vi "Striptest.vi"(1 "Simulation?":bool) -> ()   [LabVIEW 2013]
uses:
  InstrControl/SupplyControl/SupplyControl.lvclass
  InstrControl/Switching/Switching.lvclass
  InstrControl/ProbeStationControl/ProbeStationControl.lvclass
  InstrControl/LCRControl/LCRControl.lvclass
  general_VIs/globals/QC_MeasurementSetup.vi
  striptest/ProbePlan/ProbePlanParams.vi
  general_VIs/globals/QC_RunInformation.vi
  InstrControl/InstrumentSetup.vi
  <vilib>/regexp/Match Regular Expression.xnode
  InstrControl/InstrControl.lvclass
  InstrControl/ArduinoControl/ArduinoControl.lvclass
  <vilib>/Analysis/NI_AALBase.lvlib
panel:
  out "Tab Control":enum32{"Striptest Setup", "Striptest"}(tab)
  in  "Bias Voltage [V]":dbl=-150.0 format="%.1f"
  in  "Frequency [Hz] Setup":i32=500 caption="Frequency [Hz]" format="%#.3p"
  in  "Minimum fraction\nof good strips":dbl=-500.0 format="%.1g"
  in  "Quit":bool
  in  "Continue":bool
  in  "Measurement Configurations":bool
  in  "Pinholes Y/N":bool=TRUE
  in  "Capacitance Y/N":bool=TRUE
  in  "Resistance Y/N":bool=TRUE
  in  "Striptest SMU":string(combo)="Keithley 2410"
  in  "LCR Meter":string(combo)="WayneKerr 6440B"
  in  "Temperature":enum16{"Read Arduino", "Enter manually"}(ring)
  in  "Bias Supply":string(combo)="Keithley 2410"
  in  "Hardware Configurations":bool
  in  "DB Serial No. IN:":string caption="DB Serial No.:"
  in  "User:":string(combo)="Christoph"
  in  "Batch No. IN:":string caption="Batch No.:"
  in  "Device Category IN:":string(combo)="Short Strip" caption="Device Category:"
  in  "Sensor Serial No. IN:":string caption="Sensor Serial No.:"
  in  "From4":u16(ring)
  in  "From3":u16(ring)
  in  "From2":u16(ring)
  in  "From 1":u16(ring) caption="From"
  in  "To4":u16(ring)
  in  "To3":u16(ring)
  in  "To2":u16(ring)
  in  "To 1":u16(ring) caption="To"
  out "Region 1":string caption="Region"
  out "Region2":string
  out "Region3":string
  out "Region4":string
  in  "Enable1":bool
  in  "Enable4":bool
  in  "Enable2":bool
  in  "Enable3":bool
  in  "Pinhole Parameters IN":T1={"Base Voltage"=10.0, "Base Ramp [V/step]"=10.0, "Base Step [ms]"=1000, "High Voltage"=100.0, "High Ramp [V/step]"=100.0, "High Step [ms]"=1000} caption="Pinhole Measurement Parameters"
  in  "Manufacturer:":string(combo)="Hamamatsu"
  in  "Auto ReCheck":bool
  in  "Thresholds:":T2={"Current [nA]"=200.0, "Ccoupl Lo [pF/cm]"=20.0, "Ccoupl Hi [pF/cm]"=33.0, "Rbias Lo [MW]"=1.0, "Rbias Hi [MW]"=2.0}
  in  "Rolling\nCurrent Readout":bool=TRUE
  in  "settling\ndelay [ms]":i32=50
  in  "Pinhole Parameters":T1={"Base Voltage"=10.0, "Base Ramp [V/step]"=10.0, "Base Step [ms]"=1000, "High Voltage"=100.0, "High Ramp [V/step]"=100.0, "High Step [ms]"=1000}
  out "Bias On/Off:":bool
  in  "Auto quit &\nswitch off bias":bool
  out "Sensor No.:":string
  out "Device Category:":string
  out "DB Serial No.:":string
  out "Initiated:":string
  in  "ReCheck":bool
  in  "Save Data":bool
  in  "Abort":bool
  in  "Quit w/o saving":bool
  out "Probing Region:":string
  out "Probe Point:":string
  out "Current [nA]:":dbl
  out "Capacitance [pF]:":dbl
  out "Reistance [MW]:":dbl
  out "Last Probe at:":string
  out "Run Duration:":string
  out "Estimated Completion:":string
  out "Status:":string
  out "Probe Card Channels":i32=32
  in  "Show:":u16(ring)
  out "Defects":i32[][](graph)
  out "% OK:":dbl
  out "# total defects:":i32
  out "# probed":i32
  in  "Display Stats":bool=TRUE
  out "Bad Strip List":i32[](array[numeric])
  out "defect type array":i32[](array[numeric])
  out "Resistance [MW]":cluster{u32, i32, "Array OUT":dbl[]}(graph)
  out "Capacitance [pF]":cluster{u32, i32, "Array OUT":dbl[]}(graph)
  out "Current [nA]":cluster{u32, i32, "Array OUT":dbl[]}(graph)
  out "Current Reference 100V":dbl[](array[numeric])
  out "Current Reference 10V":dbl[](array[numeric])
  out "Single Needle":bool
  out "Z profile":i32[][](array[numeric])
  out "Start Temperature [°C]":dbl
  out "Last Temperature [°C]":dbl
  out "disabled channels":i32[](array[numeric])
  out "Module failed/passed":bool
  out "probe points per region":i32[](array[numeric])
  out "min scale array":i32[](array[numeric])
  out "max scale array":i32[](array[numeric])
  out "total strip number":u32
  out "Region Indices":i32[](array[numeric])
  out "Current Bias Voltage [V]":dbl
  out "Temperature Progression":T3
  # "University of \nCambridge"
  # "Sensor QC: Striptest"
  # "Current [nA]"
  # "Statistical information:"
  # "Pinholes:"
  # "Capacitance [pF]"
  # "Punchthroughs:"
  # "Shorts:"
  # "Opens:"
  # "Rpoly:"
  # "Resistance [MW]"
  # "Implant:"
  # "Current segment:"
  # "Ok  Pinhole at base  Pinhole after ramp  Short  Open  Rbias"
  # "Probe Range"
  # "Measurement Configuration"
  # "Hardware"
  # "DUT Description"
  # "Tests Included"
  # "Current status:"
  # "Measurement parameters:"
  # "DUT & Test Description:"
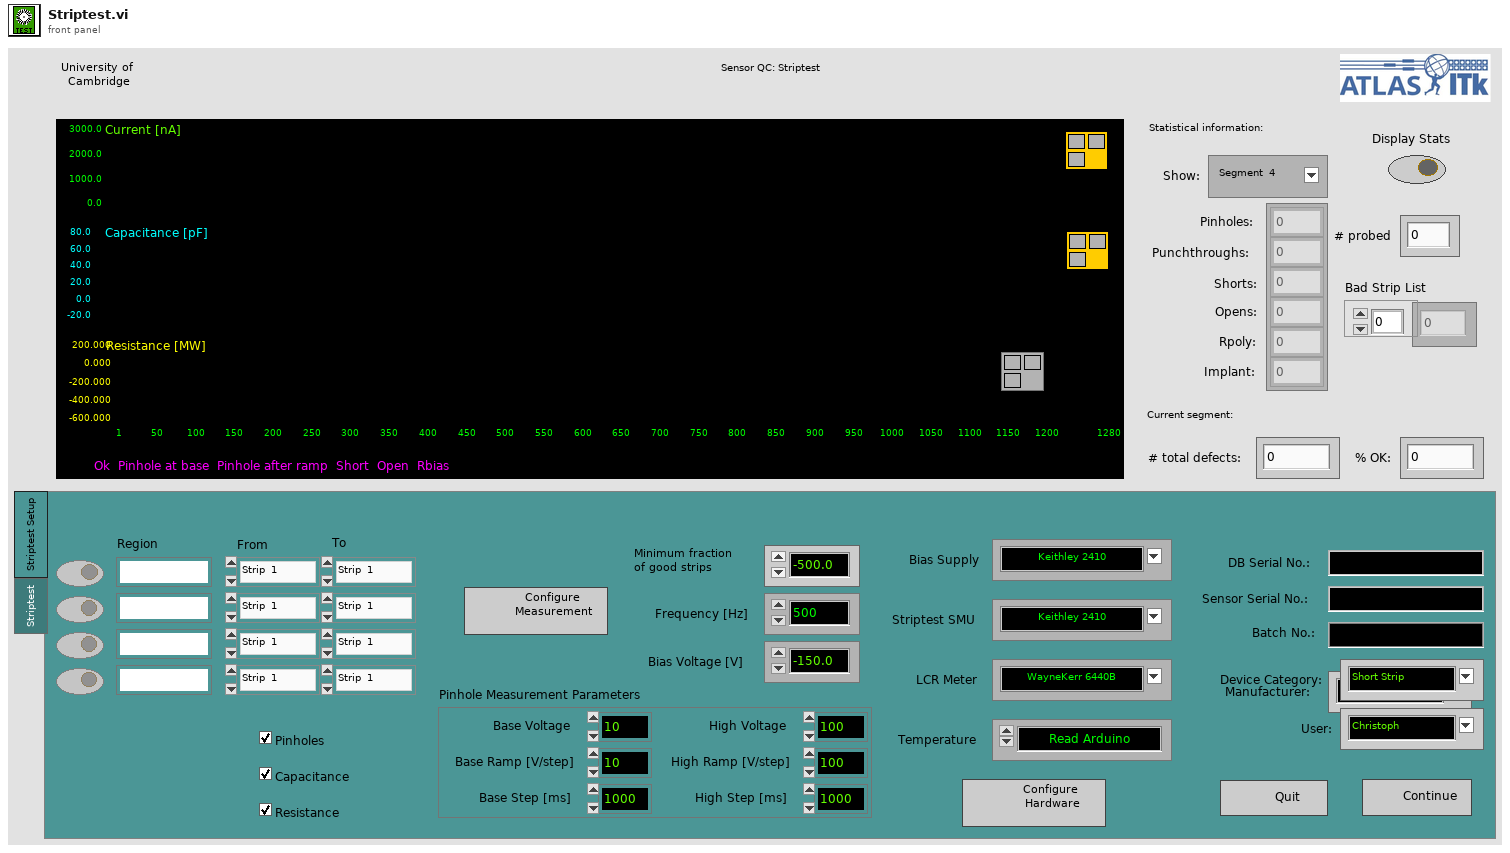
[diagram p1: front panel]
types:
  T1 = cluster{"Base Voltage":dbl, "Base Ramp [V/step]":dbl, "Base Step [ms]":i32, "High Voltage":dbl, "High Ramp [V/step]":dbl, "High Step [ms]":i32}
  T2 = cluster{"Current [nA]":dbl, "Ccoupl Lo [pF/cm]":dbl, "Ccoupl Hi [pF/cm]":dbl, "Rbias Lo [MW]":dbl, "Rbias Hi [MW]":dbl}
  T3 = cluster{"Time Array":string[], "Temperature Array [°C]":dbl[], "Humidity Array [RH %]":dbl[]}
  T4 = enum16{"Supply", "LCR", "Multimeter", "Switching"}
  T5 = enum16{"Reset", "Ground", "Striptest SMU", "Striptest LCR", "IV", "CV", "Interstrip Cap", "Interstrip Res"}
  T6 = enum16{"Reference measurement", "Baseline correcetion 10V", "Baseline correcetion 100V", "Nothing"}
  T7 = cluster{"Bias Supply":refnum<class "SupplyControl.lvclass">, "SMU":refnum<class "SupplyControl.lvclass">, "LCR":refnum<class "LCRControl.lvclass">, "Probe Card Channels":i32, "Bias Voltage [V]":dbl, "First strip":i32, "Last strip":i32, "Base Voltage [V]":dbl, "Base Ramp Step [V]":dbl, "Base Ramp Interval [ms]":u32, "High Voltage [V]":dbl, "High Ramp Step [V]":dbl, "High Ramp Interval [ms]":u32, "AC frequency [Hz]":i32, "AC amplitude [V]":dbl, "RC Configuration":u16, "Single Needle":bool, "Temperature Readout":enum16{"Read Arduino", "Enter manually"}, "Arduino":refnum<class "ArduinoControl.lvclass">, "Fraction of good strips [%]":dbl, "ProbeStation":refnum<class "ProbeStationControl.lvclass">, "Switching":refnum<class "Switching.lvclass">, "Matrix used?":bool, "Matrix X Channels":cluster{"Bias Supply / SMU LO":i32, "Bias Supply / SMU HI":i32, "CV Box LO":i32, "CV Box HI":i32, "CV Box LO IN":i32, "CV Box HI IN":i32, "Volt meter LO":i32, "Volt meter HI":i32, "Mux1 C1":i32, "Mux1 C2":i32, "Mux2 C1":i32, "Mux2 C2":i32}, "Pinholes Y/N":bool, "Capacitance Y/N":bool, "Resistance Y/N":bool, "Bias Supply Name":string, "SMU Name":string, "LCR Name":string}
  T8 = cluster{"Sensor Serial No.:":string, "Wafer Serial No.:":string, "Batch:":string, "Manufacturer:":string, "Device Category:":string, "Database Serial No.:":string, "Date Initiated:":string, "Time Initiated:":string, "Test":string, "Instruments used:":string, "Probeplan used:":string, "End of Run comment:":string, "User:":string}
  T9 = cluster{"Institute":string, "Manufacturers":string[], "Devices":string[], "Serialnumbers Lookup DB":string, "Data directory":string, "Backup & screenshot directory":string, "List of known users":string[]}
  T10 = cluster{"Strip Number OUT":i32, "X0":i32, "Y0":i32, "X1":i32, "Y1":i32, "Xref":dbl, "Yref":dbl, "ProbePlan type":u32, "Inner pads offset":ext, "Outer pads offset":ext, "l_inner":ext, "l_outer":ext, "strip numbering":u16, "Device Orientation":ext, "Stagger offset":i32, "Yoffset":dbl, "Strip pitch":dbl, "Fiducail separation":dbl, "Radius":ext, "Relative strip angles":dbl, "Probeplan description":string, "ProbePlan array":cluster{"Region":string, "ProbePoints":cluster{"X":dbl, "Y":dbl, "Label":string, "CardViable?":bool}[]}[], "Test ProbePoints":cluster{"Regions Enabled":bool[], "From index":u32[], "To index":u32[]}}
  T11 = cluster{"Region":string, "ProbePoints":cluster{"X":dbl, "Y":dbl, "Label":string, "CardViable?":bool}[]}[]
  T12 = cluster{"VISA address":refnum<visa-resource-name>, "T sensor":enum16{"SHT", "DS"}, "Arduino":refnum<class "ArduinoControl.lvclass">}
  T13 = cluster{"X":dbl, "Y":dbl, "Label":string, "CardViable?":bool}[]
  T14 = cluster{"X":dbl, "Y":dbl, "Label":string, "CardViable?":bool}
  T15 = cluster{"pass Rate in %":dbl, "Bad channel list":i32[], "No of bad strips":i32, "Defect description list":i32[], "Number of defects per category":i32[], "Defect lists":string[], "No of channels":i32, "Defect Flag array OUT":i32[][]}
  T16 = cluster{"Hi Cap":dbl, "Lo Cap":dbl, "Current threshold":dbl, "Lo R":dbl, "Hi R":dbl}
  T17 = enum16{"Reset", "Read Array", "Read Element", "Write Element", "Write Array", "Add Element", "Add Array"}
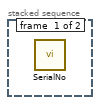
[diagram p2: hidden frame]
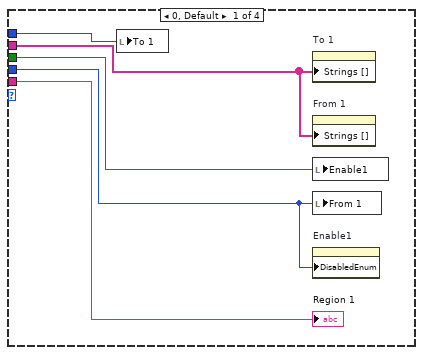
[diagram p3: hidden frame]
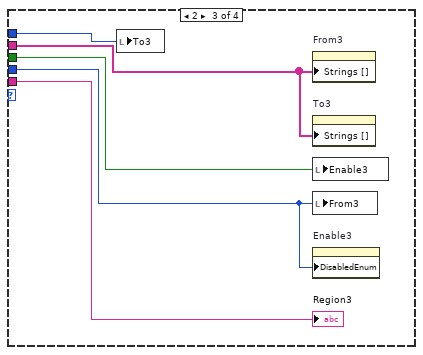
[diagram p4: hidden frame]
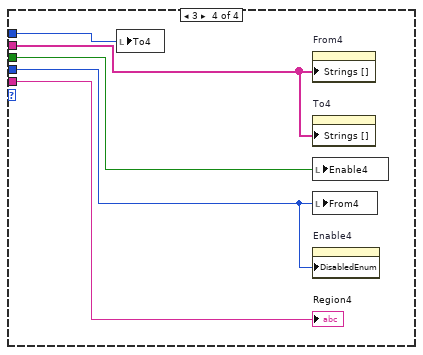
[diagram p5: hidden frame]
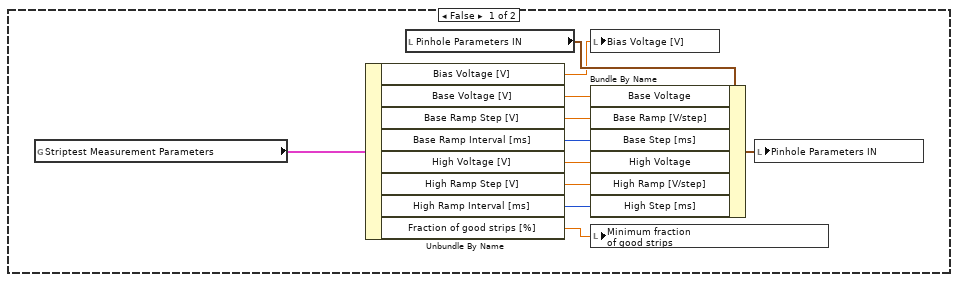
[diagram p7: hidden frame]
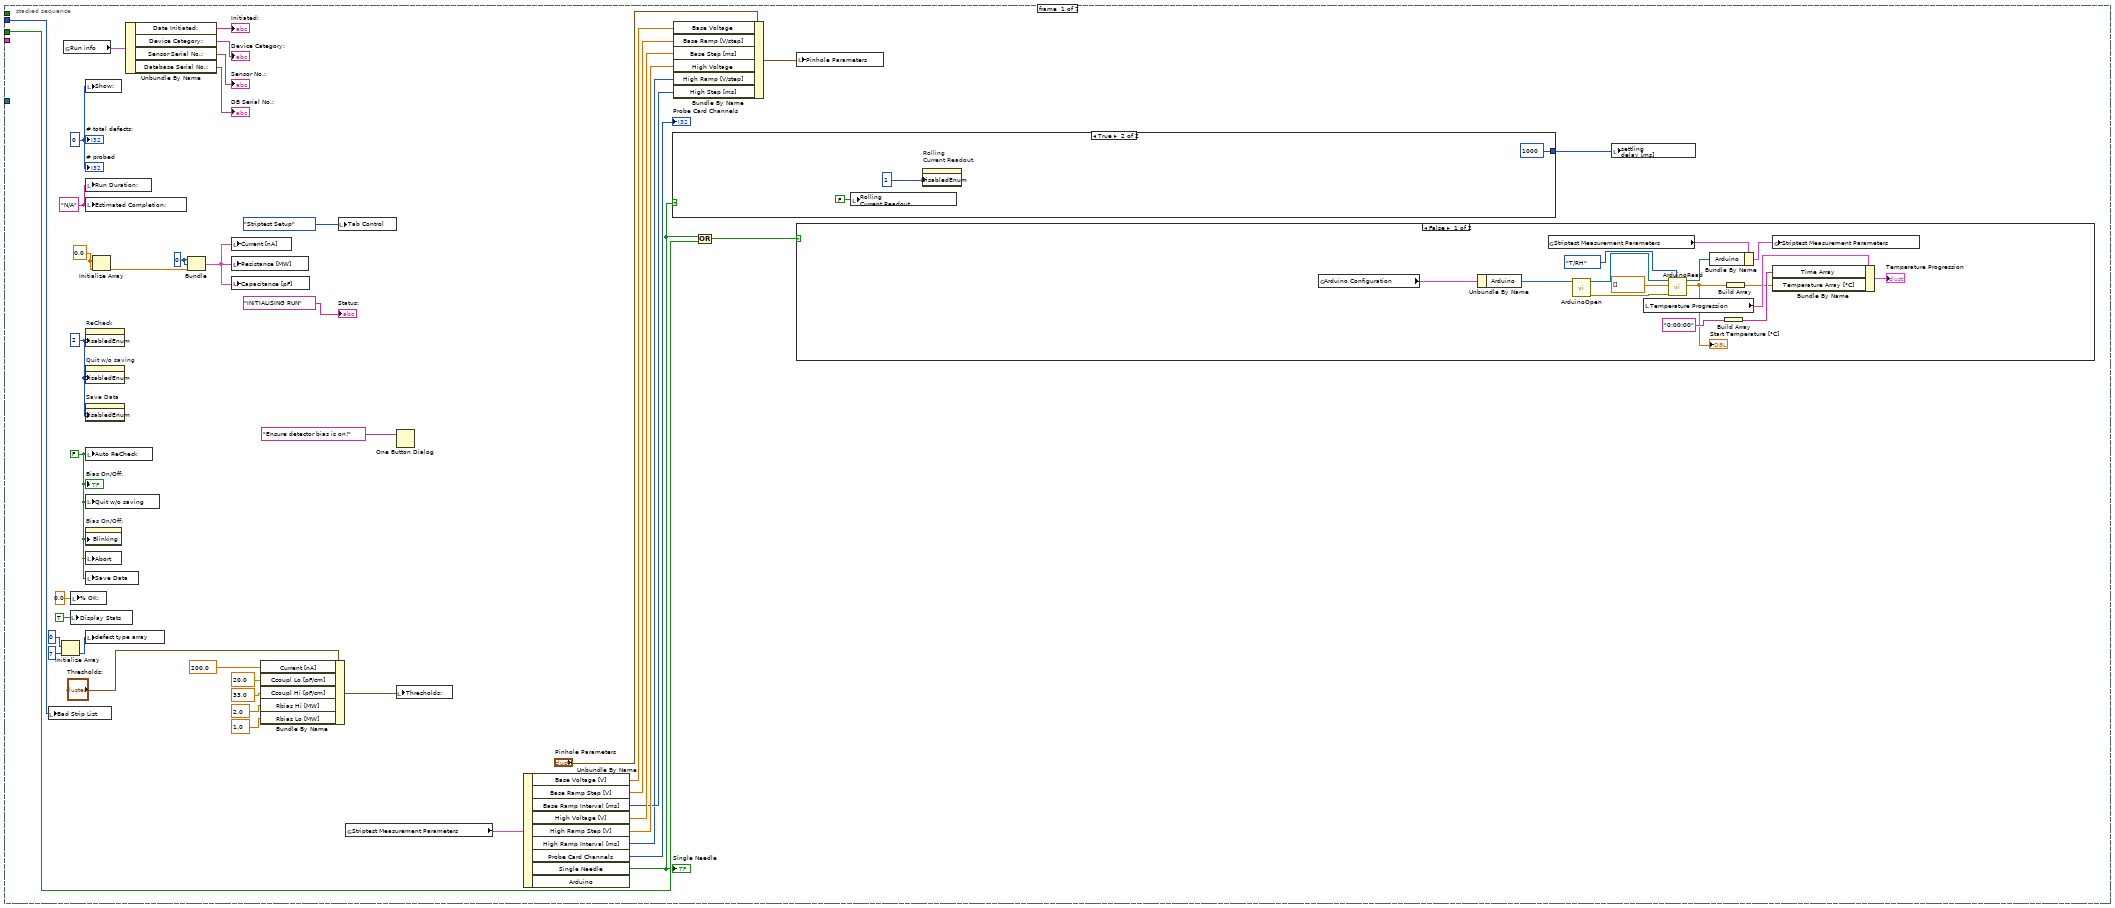
[diagram p10: hidden frame]
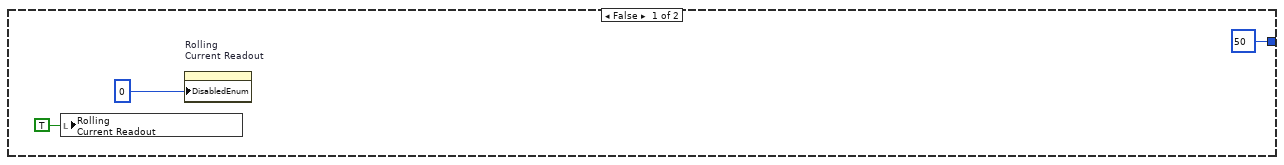
[diagram p11: hidden frame]
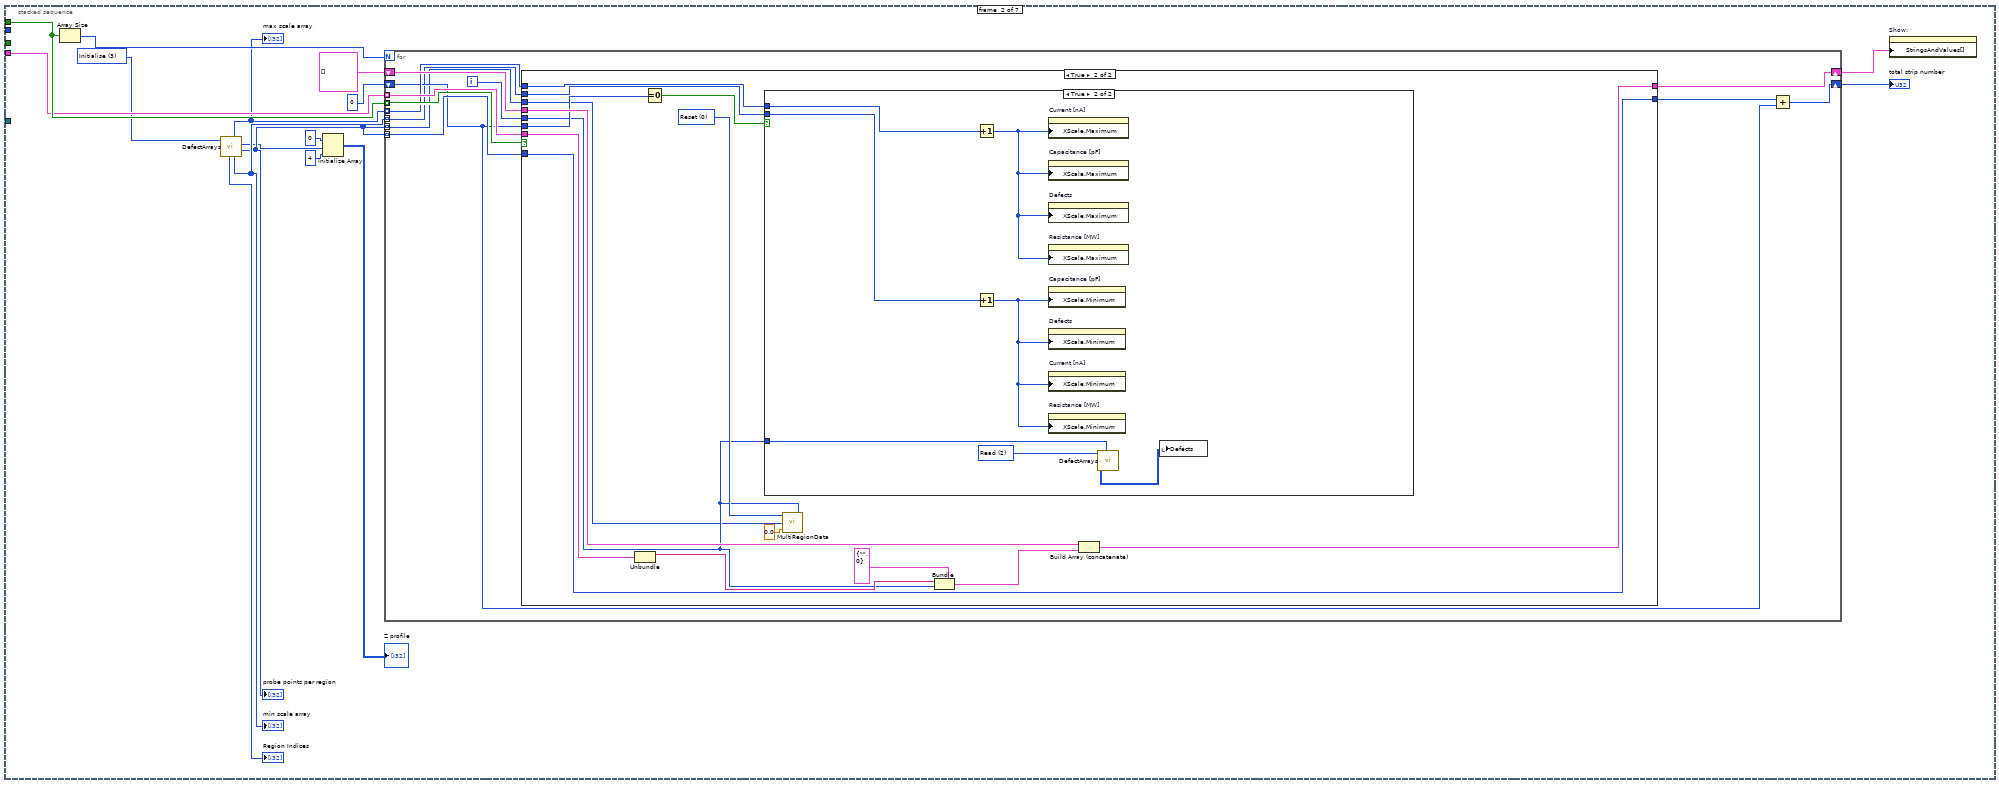
[diagram p13: hidden frame]
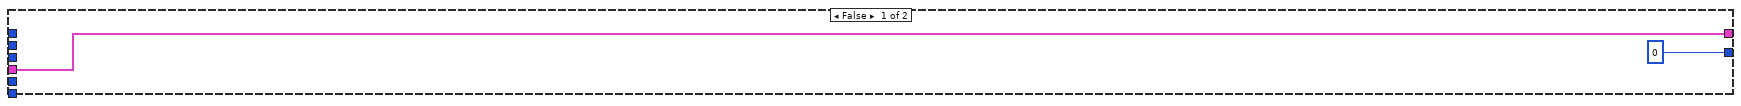
[diagram p14: hidden frame]
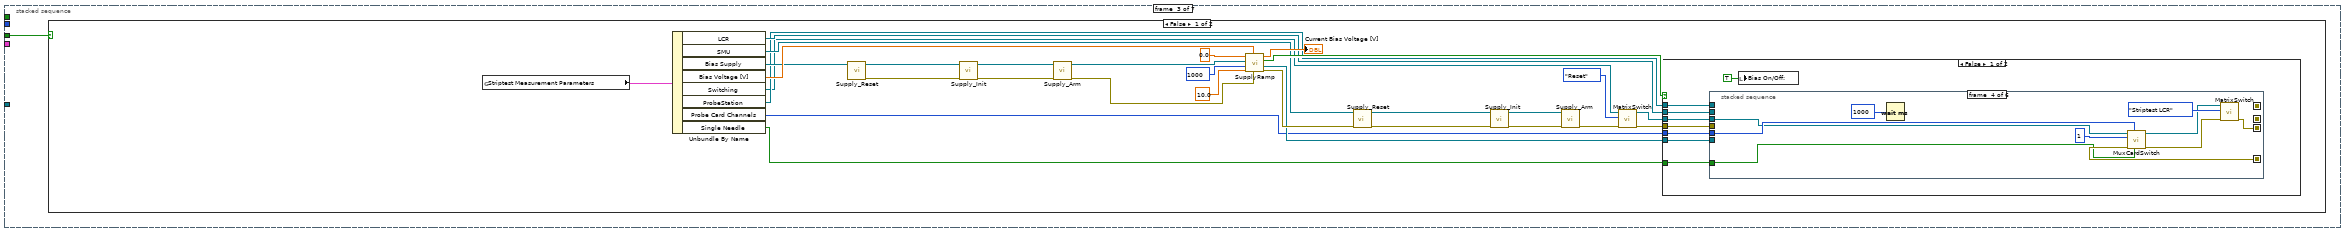
[diagram p16: hidden frame]
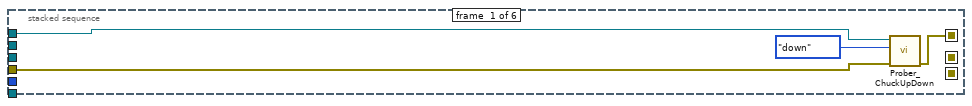
[diagram p17: hidden frame]
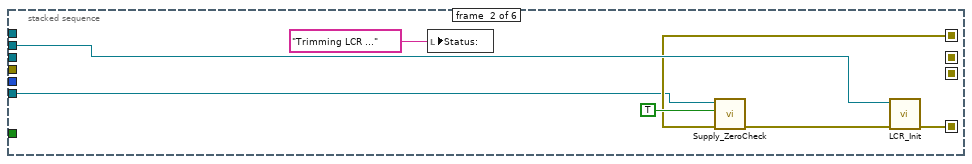
[diagram p18: hidden frame]
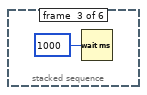
[diagram p19: hidden frame]
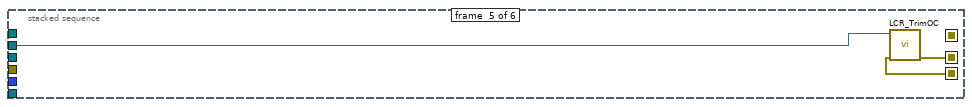
[diagram p20: hidden frame]
diagram:
  n1 = stacked-sequence {
    frame #0 {
      # "Striptest setup"
      n2 = flat-sequence {
        frame #0 {
          w1 = TRUE
          w3 = ""
          w4 = 2
          w5 = FALSE
          n3 = local write "Enable2"(w5) -> ()
          n4 = local write "Enable1"(w5) -> ()
          n5 = local write "Enable3"(w5) -> ()
          n6 = local write "Enable4"(w5) -> ()
          n7 = property on="Enable4" class="Bool (strict)"("DisabledEnum"=w4) -> ()  [unwired: 2 in, 2 out]
          n8 = property on="Enable1" class="Bool (strict)"("DisabledEnum"=w4) -> ()  [unwired: 2 in, 2 out]
          n9 = property on="Enable2" class="Bool (strict)"("DisabledEnum"=w4) -> ()  [unwired: 2 in, 2 out]
          n10 = property on="Enable3" class="Bool (strict)"("DisabledEnum"=w4) -> ()  [unwired: 2 in, 2 out]
          n11 = local write "Region 1"(w3) -> ()
          n12 = local write "Region2"(w3) -> ()
          n13 = local write "Region3"(w3) -> ()
          n14 = local write "Region4"(w3) -> ()
          n15 = call "SelectStriptestProber.vi"() -> ("error out"=w6:errorcluster, "ProbeStationControl out"=w7:refnum<class "ProbeStationControl.lvclass">)  [unwired: 10 in]
          n16 = global read "QC_MeasurementSetup.vi" "Striptest Measurement Parameters"() -> (w9:T7)
          n17 = call "InitialiseProbeplan.vi"("error in (no error)"=w6, "ProbeStationControl in"=w7) -> ()  [unwired: 8 in, 2 out]
          n18 = Bundle By Name(cluster=w9, "ProbeStation"=w7) -> (w8:T7)
          n19 = global write "QC_MeasurementSetup.vi" "Striptest Measurement Parameters"(w8) -> ()
          n20 = call "GetGlobalDefaultConfiguration.vi"("DO NOT override instruments"=w1, "Read defaults?"=w1) -> ()  [unwired: 1 in, 1 out]
          n21 = call "GetLocalConfiguration.vi"() -> ()  [unwired: 3 in, 1 out]
          "Tab Control" <- enum32{"Striptest Setup", "Striptest"}."Striptest Setup" ("Tab Control")
        }
        frame #1 {
          n22 = stacked-sequence {
            tunnel: [_ w52] -> w10
            tunnel: [_ w51] -> w11
            tunnel: [_ w50] -> w12
            tunnel: [_ w49] -> w13
            tunnel: [_ w47] -> w14
            frame #0 {
              n23 = call "SerialNo.vi"() -> ()  [unwired: 5 in, 1 out]
            }
            frame #1 {
              n24 = global read "QC_RunInformation.vi" "Run info"() -> (w48:T8)
              n25 = Unbundle By Name(w48) -> ("Sensor Serial No.:"=w52:string, "Batch:"=w51:string, "Manufacturer:"=w50:string, "Device Category:"=w49:string, "Database Serial No.:"=w47:string)
            }
          }
          n26 = global read "QC_RunInformation.vi" "Run info"() -> (w36:T8)
          n27 = Bundle By Name(cluster=w36, "Test"="Striptest") -> (w38:T8)
          n28 = call "InstrumentNames.vi"("Instrument type"=T4."Supply") -> ("error out"=w40:errorcluster, "Instrument names"=w42:string[])  [unwired: 9 in]
          n29 = property on="Bias Supply" class="CmbBox"("Strings[]"=w42) -> ()  [unwired: 2 in, 2 out]
          n30 = property on="Striptest SMU" class="CmbBox"("Strings[]"=w42) -> ()  [unwired: 2 in, 2 out]
          n31 = global write "QC_RunInformation.vi" "Run info"(w38) -> ()
          n32 = global read "QC_RunInformation.vi" "LocalConfiguration"() -> (w35:T9)
          n33 = global read "ProbePlanParams.vi" "ProbePlan Parameters IN"() -> (w46:T10)
          n34 = Unbundle By Name(w35) -> ("List of known users"=w33:string[])
          n35 = call "InstrumentNames.vi"("error in (no error)"=w40, "Instrument type"=T4."LCR") -> ("Instrument names"=w39:string[])  [unwired: 8 in, 1 out]
          n36 = global read "QC_MeasurementSetup.vi" "Striptest Measurement Parameters"() -> (w32:T7)
          n37 = local write "Sensor Serial No. IN:"(w10) -> ()
          n38 = local write "Batch No. IN:"(w11) -> ()
          n39 = local write "Manufacturer:"(w12) -> ()
          n40 = local write "Device Category IN:"(w13) -> ()
          n41 = local write "DB Serial No. IN:"(w14) -> ()
          n42 = Unbundle By Name(w46) -> ("ProbePlan array"=w45:T11)
          n43 = property on="LCR Meter" class="CmbBox"("Strings[]"=w39) -> ()  [unwired: 2 in, 2 out]
          n44 = property on="User:" class="CmbBox"("Strings[]"=w33, "AllowUndefStrs"=TRUE) -> ()  [unwired: 2 in, 2 out]
          n45 = Array Size(array=w45) -> (size(s)=w44:i32)
          n46 = for {
            N: w44 -> [_]
            tunnel: w45 -> [w54]
            tunnel: w45 -> [w58] mode=indexing
            i -> [w61]
            n47 = Unbundle(w58) -> ("Region"=w57:string)  [unwired: 1 out]
            n48 = call "GetLabels.vi"("Array"=w54) -> ("Strip Labels"=w53:string[])  [unwired: 3 out]
            n49 = Array Size(array=w53) -> (size(s)=w56:i32)
            n50 = Decrement(x=w56) -> (x-1=w55:i32)
            n51 = case shown="1" w61 {
              tunnel: TRUE -> [w66 w70 w76 w81]
              tunnel: 0 -> [w62 w68 w72 w78]
              tunnel: w57 -> [w64 w69 w74 w79]
              tunnel: w53 -> [w63 w67 w73 w77]
              tunnel: w55 -> [w65 w71 w75 w80]
              frame 0, Default {
                n52 = local write "To 1"(w65) -> ()
                n53 = property on="To 1" class="Ring (strict)"("Strings []"=w63) -> ()  [unwired: 2 in, 2 out]
                n54 = property on="From 1" class="Ring (strict)"("Strings []"=w63) -> ()  [unwired: 2 in, 2 out]
                n55 = local write "Enable1"(w66) -> ()
                n56 = local write "From 1"(w62) -> ()
                n57 = property on="Enable1" class="Bool (strict)"("DisabledEnum"=w62) -> ()  [unwired: 2 in, 2 out]
                "Region 1" <- w64
              }
              frame 1 {
                n58 = local write "To2"(w71) -> ()
                n59 = property on="From2" class="Ring (strict)"("Strings []"=w67) -> ()  [unwired: 2 in, 2 out]
                n60 = property on="To2" class="Ring (strict)"("Strings []"=w67) -> ()  [unwired: 2 in, 2 out]
                n61 = local write "Enable2"(w70) -> ()
                n62 = local write "From2"(w68) -> ()
                n63 = property on="Enable2" class="Bool (strict)"("DisabledEnum"=w68) -> ()  [unwired: 2 in, 2 out]
                "Region2" <- w69
              }
              frame 2 {
                n64 = local write "To3"(w75) -> ()
                n65 = property on="From3" class="Ring (strict)"("Strings []"=w73) -> ()  [unwired: 2 in, 2 out]
                n66 = property on="To3" class="Ring (strict)"("Strings []"=w73) -> ()  [unwired: 2 in, 2 out]
                n67 = local write "Enable3"(w76) -> ()
                n68 = local write "From3"(w72) -> ()
                n69 = property on="Enable3" class="Bool (strict)"("DisabledEnum"=w72) -> ()  [unwired: 2 in, 2 out]
                "Region3" <- w74
              }
              frame 3 {
                n70 = local write "To4"(w80) -> ()
                n71 = property on="From4" class="Ring (strict)"("Strings []"=w77) -> ()  [unwired: 2 in, 2 out]
                n72 = property on="To4" class="Ring (strict)"("Strings []"=w77) -> ()  [unwired: 2 in, 2 out]
                n73 = local write "Enable4"(w81) -> ()
                n74 = local write "From4"(w78) -> ()
                n75 = property on="Enable4" class="Bool (strict)"("DisabledEnum"=w78) -> ()  [unwired: 2 in, 2 out]
                "Region4" <- w79
              }
            }
          }
          n76 = Unbundle By Name(w32) -> ("Probe Card Channels"=w31:i32, "Bias Voltage [V]"=w22:dbl, "Base Voltage [V]"=w28:dbl, "Base Ramp Step [V]"=w27:dbl, "Base Ramp Interval [ms]"=w26:u32, "High Voltage [V]"=w25:dbl, "High Ramp Step [V]"=w24:dbl, "High Ramp Interval [ms]"=w23:u32, "Single Needle"=w21:bool, "Temperature Readout"=w20:enum16{"Read Arduino", "Enter manually"}, "Fraction of good strips [%]"=w19:dbl, "AC frequency [Hz]"=w18:i32, "Pinholes Y/N"=w17:bool, "Capacitance Y/N"=w16:bool, "Resistance Y/N"=w15:bool)
          n77 = local read "Pinhole Parameters IN"() -> (w30:T1)
          n78 = Bundle By Name(cluster=w30, "Base Voltage"=w28, "Base Ramp [V/step]"=w27, "Base Step [ms]"=w26, "High Voltage"=w25, "High Ramp [V/step]"=w24, "High Step [ms]"=w23) -> (w29:T1)
          n79 = local write "Probe Card Channels"(w31) -> ()
          n80 = local write "Bias Voltage [V]"(w22) -> ()
          n81 = local write "Single Needle"(w21) -> ()
          n82 = local write "Temperature"(w20) -> ()
          n83 = local write "Minimum fraction\nof good strips"(w19) -> ()
          n84 = local write "Frequency [Hz] Setup"(w18) -> ()
          n85 = local write "Pinholes Y/N"(w17) -> ()
          n86 = local write "Capacitance Y/N"(w16) -> ()
          n87 = local write "Resistance Y/N"(w15) -> ()
          n88 = local write "Pinhole Parameters IN"(w29) -> ()
        }
        frame #2 {
          n89 = while {
            shift-right: [w85] -> _
            shift-left: FALSE -> [w87]
            stop <- "Continue" stop-if-true
            n90 = Stop(stop? (T)="Quit") -> ()
            n91 = local read "Sensor Serial No. IN:"() -> (w93:string)
            n92 = local read "DB Serial No. IN:"() -> (w91:string)
            n93 = local read "Batch No. IN:"() -> (w92:string)
            n94 = Empty String/Path?(string/path=w93) -> (empty?=w90:bool)
            n95 = Empty String/Path?(string/path=w92) -> (empty?=w89:bool)
            n96 = Empty String/Path?(string/path=w91) -> (empty?=w88:bool)
            n97 = case shown="True" "Measurement Configurations" {
              frame False {
              }
              frame True {
                n98 = Two Button Dialog(message="With this, you will change QC measurement parameters defined by the collaboration!\n\nDo you really wish to continue?", 2:"YES") -> (T button?=w99:bool)  [unwired: 1 in]
                n99 = case shown="True" w99 {
                  frame False {
                    n100 = global read "QC_MeasurementSetup.vi" "Striptest Measurement Parameters"() -> (w112:T7)
                    n101 = Unbundle By Name(w112) -> ("Bias Voltage [V]"=w102:dbl, "Base Voltage [V]"=w109:dbl, "Base Ramp Step [V]"=w108:dbl, "Base Ramp Interval [ms]"=w107:u32, "High Voltage [V]"=w106:dbl, "High Ramp Step [V]"=w105:dbl, "High Ramp Interval [ms]"=w104:u32, "Fraction of good strips [%]"=w103:dbl)
                    n102 = local read "Pinhole Parameters IN"() -> (w111:T1)
                    n103 = local write "Bias Voltage [V]"(w102) -> ()
                    n104 = Bundle By Name(cluster=w111, "Base Voltage"=w109, "Base Ramp [V/step]"=w108, "Base Step [ms]"=w107, "High Voltage"=w106, "High Ramp [V/step]"=w105, "High Step [ms]"=w104) -> (w110:T1)
                    n105 = local write "Minimum fraction\nof good strips"(w103) -> ()
                    n106 = local write "Pinhole Parameters IN"(w110) -> ()
                  }
                  frame True {
                    n107 = global read "QC_MeasurementSetup.vi" "Striptest Measurement Parameters"() -> (w123:T7)
                    n108 = Unbundle By Name("Pinhole Parameters IN") -> ("Base Voltage"=w119:dbl, "Base Ramp [V/step]"=w118:dbl, "Base Step [ms]"=w117:i32, "High Voltage"=w116:dbl, "High Ramp [V/step]"=w115:dbl, "High Step [ms]"=w114:i32)
                    n109 = Bundle By Name(cluster=w123, "Bias Voltage [V]"="Bias Voltage [V]", "Base Voltage [V]"=w119, "Base Ramp Step [V]"=w118, "Base Ramp Interval [ms]"=w117, "High Voltage [V]"=w116, "High Ramp Step [V]"=w115, "High Ramp Interval [ms]"=w114, "Fraction of good strips [%]"="Minimum fraction\nof good strips") -> (w122:T7)
                    n110 = global write "QC_MeasurementSetup.vi" "Striptest Measurement Parameters"(w122) -> ()
                  }
                }
              }
            }
            n111 = case shown="True" "Hardware Configurations" {
              tunnel: [w124 w125] -> w85
              tunnel: w87 -> [w124 _]
              frame False {
              }
              frame True {
                n112 = call "HardwareConfiguration.vi"() -> ("configured?"=w125:bool)  [unwired: 11 in]
              }
            }
            n113 = Compound Arithmetic op=OR(w90, w89, w88) -> (invert w94:bool)
            n114 = Select(t=0, s=w94, f=2) -> (s? t:f=w84:i32)
            n115 = property on="Continue" class="Bool"("DisabledEnum"=w84) -> ()  [unwired: 2 in, 2 out]
          }
        }
        frame #3 {
          w146 = TRUE
          w153 = T4."Supply" ("Instrument type")
          n116 = call "InstrumentSelection.vi"("Verify GPIB address"=w146, "Instrument type"=w153, "Instrument name IN"="Bias Supply") -> ("error out"=w159:errorcluster, "Instrument name OUT"=w133:string, "Supply"=w154:refnum<class "SupplyControl.lvclass">)  [unwired: 3 in, 3 out]
          n117 = call "InstrumentSelection.vi"("error in (no error)"=w159, "Verify GPIB address"=w146, "Instrument type"=w153, "Instrument name IN"="Striptest SMU") -> ("error out"=w147:errorcluster, "Instrument name OUT"=w132:string, "Supply"=w151:refnum<class "SupplyControl.lvclass">)  [unwired: 2 in, 3 out]
          n118 = global read "ProbePlanParams.vi" "ProbePlan Parameters IN"() -> (w182:T10)
          n119 = Build Array("Enable1", "Enable2", "Enable3", "Enable4") -> (w180:bool[])
          n120 = Build Array("From 1", "From2", "From3", "From4") -> (w179:u16[])
          n121 = Build Array("To 1", "To2", "To3", "To4") -> (w178:u16[])
          n122 = call "InstrumentSelection.vi"("error in (no error)"=w147, "Verify GPIB address"=w146, "Instrument type"=T4."LCR", "Instrument name IN"="LCR Meter") -> ("error out"=w148:errorcluster, "Instrument name OUT"=w131:string, "LCR"=w150:refnum<class "LCRControl.lvclass">)  [unwired: 2 in, 3 out]
          n123 = global read "QC_MeasurementSetup.vi" "Striptest Measurement Parameters"() -> (w156:T7)
          n124 = Bundle By Name(cluster=w182, "Test ProbePoints.Regions Enabled"=w180, "Test ProbePoints.From index"=w179, "Test ProbePoints.To index"=w178) -> (w181:T10)
          n125 = Unbundle By Name(w182) -> ("Probeplan description"=w137:string)
          n126 = Format Into String(format string="%s, %s, %s", w133, w132, w131) -> (resulting string=w130:string)  [unwired: 2 in, 1 out]
          n127 = call "InstrumentSelection.vi"("error in (no error)"=w148, "Verify GPIB address"=w146, "Instrument type"=T4."Switching", "Instrument name IN"="Pickering Matrix") -> ("Switching"=w149:refnum<class "Switching.lvclass">)  [unwired: 2 in, 5 out]
          n128 = global read "QC_RunInformation.vi" "Run info"() -> (w157:T8)
          n129 = Get Date/Time String(date format (0)=enum16{"short", "long", "abbreviated"}."abbreviated", want seconds? (F)=TRUE) -> (date string=w139:string, time string=w138:string)  [unwired: 1 in]
          n130 = Bundle By Name(cluster=w156, "Bias Supply"=w154, "SMU"=w151, "LCR"=w150, "Switching"=w149, "Temperature Readout"="Temperature", "AC frequency [Hz]"="Frequency [Hz] Setup", "Pinholes Y/N"="Pinholes Y/N", "Capacitance Y/N"="Capacitance Y/N", "Resistance Y/N"="Resistance Y/N") -> (w155:T7)
          n131 = global write "ProbePlanParams.vi" "ProbePlan Parameters IN"(w181) -> ()
          n132 = global write "QC_MeasurementSetup.vi" "Striptest Measurement Parameters"(w155) -> ()
          n133 = Bundle By Name(cluster=w157, "Sensor Serial No.:"="Sensor Serial No. IN:", "Batch:"="Batch No. IN:", "Manufacturer:"="Manufacturer:", "Device Category:"="Device Category IN:", "Database Serial No.:"="DB Serial No. IN:", "Date Initiated:"=w139, "Time Initiated:"=w138, "Instruments used:"=w130, "Probeplan used:"=w137, "User:"="User:") -> (w165:T8)
          n134 = global write "QC_RunInformation.vi" "Run info"(w165) -> ()
        }
      }
    }
    frame #1 {
      # "Striptest measurement procedure"
      n135 = global read "QC_MeasurementSetup.vi" "Striptest Measurement Parameters"() -> (w183:T7)
      n136 = global read "ProbePlanParams.vi" "ProbePlan Parameters IN"() -> (w190:T10)
      n137 = Unbundle By Name(w190) -> ("Test ProbePoints.Regions Enabled"=w186:bool[], "ProbePlan array"=w185:T11)
      n138 = Unbundle By Name(w183) -> ("ProbeStation"=w184:refnum<class "ProbeStationControl.lvclass">)
      n139 = Initialize Array(0) -> (w188:i32[])  [unwired: 1 in]
      n140 = stacked-sequence {
        tunnel: w188 -> [w212 _ _ _ w414 _ _]
        tunnel: "Simulation?" -> [w206 _ w307 w392 _ w1033 w1090]
        tunnel: w186 -> [_ w269 _ _ w417 _ w1089]
        tunnel: w185 -> [_ w268 _ _ w415 _ _]
        tunnel: w184 -> [_ _ _ w390 _ w1032 _]
        frame #0 {
          w214 = "N/A"
          w209 = FALSE
          w222 = 2
          w215 = 0
          w232 = 0
          w231 = 0.0
          n141 = local write "Bad Strip List"(w212) -> ()
          n142 = Initialize Array(0, 7 ("Dimension Size")) -> (w210:i32[])
          n143 = global read "QC_RunInformation.vi" "Run info"() -> (w229:T8)
          n144 = local write "Display Stats"(TRUE) -> ()
          n145 = local write "% OK:"(0.0) -> ()
          n146 = local write "Show:"(w215) -> ()
          n147 = local write "Run Duration:"(w214) -> ()
          n148 = local write "Estimated Completion:"(w214) -> ()
          n149 = property on="ReCheck" class="Bool"("DisabledEnum"=w222) -> ()  [unwired: 2 in, 2 out]
          n150 = property on="Quit w/o saving" class="Bool (strict)"("DisabledEnum"=w222) -> ()  [unwired: 2 in, 2 out]
          n151 = property on="Save Data" class="Bool (strict)"("DisabledEnum"=w222) -> ()  [unwired: 2 in, 2 out]
          n152 = local write "Auto ReCheck"(w209) -> ()
          n153 = local write "Quit w/o saving"(w209) -> ()
          n154 = property on="Bias On/Off:" class="Bool (strict)"("Blinking"=w209) -> ()  [unwired: 2 in, 2 out]
          n155 = local write "Abort"(w209) -> ()
          n156 = local write "Save Data"(w209) -> ()
          n157 = local write "defect type array"(w210) -> ()
          n158 = Initialize Array(w231, w231) -> (w233:dbl[])
          n159 = Unbundle By Name(w229) -> ("Date Initiated:"=→"Initiated:":string, "Device Category:"=→"Device Category:":string, "Sensor Serial No.:"=→"Sensor No.:":string, "Database Serial No.:"=→"DB Serial No.:":string)
          n160 = Bundle(w232, w232, w233) -> (w230:cluster{i32, i32, dbl[]})  [unwired: 1 in]
          n161 = local write "Current [nA]"(w230) -> ()
          n162 = local write "Resistance [MW]"(w230) -> ()
          n163 = local write "Capacitance [pF]"(w230) -> ()
          n164 = Bundle By Name(cluster="Thresholds:", "Current [nA]"=200.0 ("CapLo"), "Ccoupl Lo [pF/cm]"=20.0 ("CapLo"), "Ccoupl Hi [pF/cm]"=33.0 ("CapHi"), "Rbias Hi [MW]"=2.0 ("Rpolyhi"), "Rbias Lo [MW]"=1.0 ("RpolyLo")) -> (w220:T2)
          n165 = local write "Tab Control"(enum32{"Striptest Setup", "Striptest"}."Striptest Setup" ("Tab Control")) -> ()
          n166 = global read "QC_MeasurementSetup.vi" "Striptest Measurement Parameters"() -> (w194:T7)
          n167 = One Button Dialog(message="Ensure detector bias is on!") -> ()  [unwired: 1 in, 1 out]
          n168 = local write "Thresholds:"(w220) -> ()
          n169 = Unbundle By Name(w194) -> ("Base Voltage [V]"=w202:dbl, "Base Ramp Step [V]"=w203:dbl, "Base Ramp Interval [ms]"=w199:u32, "High Voltage [V]"=w200:dbl, "High Ramp Step [V]"=w201:dbl, "High Ramp Interval [ms]"=w198:u32, "Probe Card Channels"=→"Probe Card Channels":i32, "Single Needle"=w193:bool)  [unwired: 1 out]
          "Single Needle" <- w193
          n170 = case shown="True" w193 {
            tunnel: [50 1000] -> w195
            frame False {
              n171 = local write "Rolling\nCurrent Readout"(TRUE) -> ()
              n172 = property on="Rolling\nCurrent Readout" class="Bool (strict)"("DisabledEnum"=0) -> ()  [unwired: 2 in, 2 out]
            }
            frame True {
              n173 = local write "Rolling\nCurrent Readout"(FALSE) -> ()
              n174 = property on="Rolling\nCurrent Readout" class="Bool (strict)"("DisabledEnum"=1) -> ()  [unwired: 2 in, 2 out]
            }
          }
          n175 = Bundle By Name(cluster="Pinhole Parameters", "Base Voltage"=w202, "Base Ramp [V/step]"=w203, "Base Step [ms]"=w200, "High Voltage"=w201, "High Ramp [V/step]"=w198, "High Step [ms]"=w199) -> (w204:T1)
          n176 = Or(x=w193, y=w206) -> (x .or. y?=w205:bool)
          n177 = local write "Pinhole Parameters"(w204) -> ()
          n178 = case shown="False" w205 {
            frame False {
              n179 = global read "InstrumentSetup.vi" "Arduino Configuration"() -> (w254:T12)
              n180 = Unbundle By Name(w254) -> ("Arduino"=w246:refnum<class "ArduinoControl.lvclass">)
              n181 = global read "QC_MeasurementSetup.vi" "Striptest Measurement Parameters"() -> (w242:T7)
              n182 = call "ArduinoOpen.vi"("ArduinoControl in"=w246) -> ("error out"=w244:errorcluster, "ArduinoControl out"=w245:refnum<class "ArduinoControl.lvclass">)  [unwired: 9 in]
              n183 = local read "Temperature Progression"() -> (w253:T3)
              n184 = call "ArduinoRead.vi"("Arduino function"=enum16{"T/RH", "Interlock", "Edgesense"}."T/RH", "error in (no error)"=w244, "Temperature IN"=dbl[] [], "ArduinoControl in"=w245) -> ("Temperature [°C]"=w248:dbl, "ArduinoControl out"=w240:refnum<class "ArduinoControl.lvclass">)  [unwired: 2 in, 4 out]
              "Start Temperature [°C]" <- w248
              n185 = Bundle By Name(cluster=w242, "Arduino"=w240) -> (w241:T7)
              n186 = Build Array("0:00:00") -> (w249:string[])
              n187 = Build Array(w248) -> (w247:dbl[])
              n188 = global write "QC_MeasurementSetup.vi" "Striptest Measurement Parameters"(w241) -> ()
              n189 = Bundle By Name(cluster=w253, "Time Array"=w249, "Temperature Array [°C]"=w247) -> (→"Temperature Progression":T3)
            }
            frame True {
            }
          }
          n190 = local write "settling\ndelay [ms]"(w195) -> ()
          "# total defects:" <- w215
          "# probed" <- w215
          "Status:" <- "INITIALISING RUN"
          "Bias On/Off:" <- w209
        }
        frame #1 {
          w264 = u16 3 items=["Nothing", "Write", "Read", "Initialise"] ("action")
          n191 = Array Size(array=w269) -> (size(s)=w270:i32)
          n192 = call "DefectArrays.vi"("action"=w264) -> ("Region Indices"=→"Region Indices":i32[], "To"=w263:i32[], "max. No. of points in region"=w255:i32, "From"=w262:i32[], "No. of points in region"=w257:i32[])  [unwired: 2 in, 3 out]
          "max scale array" <- w263
          "min scale array" <- w262
          "probe points per region" <- w257
          n193 = Initialize Array(0, w255, 4) -> (→"Z profile":i32[][])
          n194 = for {
            N: w270 -> [_]
            tunnel: w269 -> [w282] mode=indexing
            shift-right: [w281] -> w267
            shift-left: cluster{string, i32}[] [] -> [w280]
            tunnel: w268 -> [w279] mode=indexing
            tunnel: w257 -> [w274] mode=indexing
            tunnel: w263 -> [w275] mode=indexing
            tunnel: w262 -> [w272] mode=indexing
            shift-right: [w276] -> w266
            shift-left: 0 -> [w273]
            tunnel: w257 -> [w271] mode=indexing
            i -> [w277]
            n195 = case shown="True" w282 {
              tunnel: w280 -> [w283 w298]
              tunnel: [w283 w297] -> w281
              tunnel: w279 -> [_ w299]
              tunnel: [0 w293] -> w278
              tunnel: w277 -> [_ w288]
              tunnel: w275 -> [_ w295]
              tunnel: w272 -> [_ w294]
              tunnel: w274 -> [_ w293]
              tunnel: w273 -> [_ w292]
              tunnel: w271 -> [_ w286]
              frame False {
              }
              frame True {
                w290 = u32 0 items=["Reset", "Read Array", "Read Element", "Write Element", "Write Array"] ("Action")
                n196 = Unbundle(w299) -> ("Region"=w289:string)  [unwired: 1 out]
                n197 = Equal To 0?(x=w292) -> (x = 0?=w296:bool)
                n198 = case shown="True" w296 {
                  tunnel: w295 -> [_ w301]
                  tunnel: w294 -> [_ w303]
                  tunnel: w288 -> [_ w304]
                  frame False {
                  }
                  frame True {
                    w306 = u16 2 items=["Nothing", "Write", "Read", "Initialise"] ("action")
                    n199 = Increment(x=w301) -> (x+1=w300:i32)
                    n200 = Increment(x=w303) -> (x+1=w302:i32)
                    n201 = property on="Current [nA]" class="WFGraph (strict)"("XScale.Maximum"=w300) -> ()  [unwired: 2 in, 2 out]
                    n202 = property on="Capacitance [pF]" class="WFGraph (strict)"("XScale.Maximum"=w300) -> ()  [unwired: 2 in, 2 out]
                    n203 = property on="Defects" class="IntGraph (strict)"("XScale.Maximum"=w300) -> ()  [unwired: 2 in, 2 out]
                    n204 = property on="Resistance [MW]" class="WFGraph (strict)"("XScale.Maximum"=w300) -> ()  [unwired: 2 in, 2 out]
                    n205 = property on="Capacitance [pF]" class="WFGraph (strict)"("XScale.Minimum"=w302) -> ()  [unwired: 2 in, 2 out]
                    n206 = property on="Defects" class="IntGraph (strict)"("XScale.Minimum"=w302) -> ()  [unwired: 2 in, 2 out]
                    n207 = property on="Current [nA]" class="WFGraph (strict)"("XScale.Minimum"=w302) -> ()  [unwired: 2 in, 2 out]
                    n208 = property on="Resistance [MW]" class="WFGraph (strict)"("XScale.Minimum"=w302) -> ()  [unwired: 2 in, 2 out]
                    n209 = call "DefectArrays.vi"("action"=w306, "Region Index"=w304) -> ("Defect array OUT"=w305:i32[][])  [unwired: 1 in, 7 out]
                    n210 = local write "Defects"(w305) -> ()
                  }
                }
                n211 = call "MultiRegionData.vi"("Action"=w290, "Array Size / Index"=w286, "Data IN"=0.0, "Region index"=w288) -> ()  [unwired: 2 in, 2 out]
                n212 = Bundle(cluster=cluster{string, i32} {"", 0}, w289, w288) -> (w287:cluster{string, i32})
                n213 = Build Array (concatenate)(w298, w287) -> (w297:cluster{string, i32}[])
              }
            }
            n214 = Add(x=w278, y=w273) -> (x+y=w276:i32)
          }
          "total strip number" <- w266
          n215 = property on="Show:" class="Ring (strict)"("StringsAndValues[]"=w267) -> ()  [unwired: 2 in, 2 out]
        }
        frame #2 {
          n216 = case shown="False" w307 {
            frame False {
              n217 = global read "QC_MeasurementSetup.vi" "Striptest Measurement Parameters"() -> (w336:T7)
              n218 = Unbundle By Name(w336) -> ("LCR"=w313:refnum<class "LCRControl.lvclass">, "SMU"=w314:refnum<class "SupplyControl.lvclass">, "Bias Supply"=w315:refnum<class "SupplyControl.lvclass">, "Bias Voltage [V]"=w325:dbl, "Switching"=w310:refnum<class "Switching.lvclass">, "ProbeStation"=w312:refnum<class "ProbeStationControl.lvclass">, "Probe Card Channels"=w309:i32, "Single Needle"=w308:bool)
              n219 = call-dynamic "Supply_Reset.vi"("SupplyControl in"=w315) -> ("error out"=w329:errorcluster, "SupplyControl out"=w332:refnum<class "SupplyControl.lvclass">)  [unwired: 9 in]
              n220 = call-dynamic "Supply_Init.vi"("error in (no error)"=w329, "SupplyControl in"=w332) -> ("error out"=w330:errorcluster, "SupplyControl out"=w331:refnum<class "SupplyControl.lvclass">)  [unwired: 8 in]
              n221 = call-dynamic "Supply_Arm.vi"("error in (no error)"=w330, "SupplyControl in"=w331) -> ("error out"=w327:errorcluster, "SupplyControl out"=w328:refnum<class "SupplyControl.lvclass">)  [unwired: 8 in]
              n222 = call "SupplyRamp.vi"("error in"=w327, "Requested Voltage"=w325, "Step Size"=10.0, "Step Delay"=1000, "Supply IN"=w328, "Starting Voltage"=0.0) -> ("error out"=w326:errorcluster, "Supply OUT"=w311:refnum<class "SupplyControl.lvclass">, "Compliance exceeded"=w319:bool, "Current Voltage"=→"Current Bias Voltage [V]":dbl)  [unwired: 2 in]
              n223 = call-dynamic "Supply_Reset.vi"("error in (no error)"=w326, "SupplyControl in"=w314) -> ("error out"=w323:errorcluster, "SupplyControl out"=w322:refnum<class "SupplyControl.lvclass">)  [unwired: 8 in]
              n224 = call-dynamic "Supply_Init.vi"("error in (no error)"=w323, "SupplyControl in"=w322) -> ("error out"=w324:errorcluster, "SupplyControl out"=w321:refnum<class "SupplyControl.lvclass">)  [unwired: 8 in]
              n225 = call-dynamic "Supply_Arm.vi"("error in (no error)"=w324, "SupplyControl in"=w321) -> ("error out"=w337:errorcluster)  [unwired: 8 in, 1 out]
              n226 = call-dynamic "MatrixSwitch.vi"("error in (no error)"=w337, "Action"=T5."Reset", "Switching in"=w310) -> ("error out"=w316:errorcluster, "Switching out"=w317:refnum<class "Switching.lvclass">)  [unwired: 6 in, 1 out]
              n227 = case shown="False" w319 {
                selector: w319 -> [_ w389]
                tunnel: w317 -> [w344 _]
                tunnel: w316 -> [w343 _]
                tunnel: w313 -> [w342 _]
                tunnel: w312 -> [w341 _]
                tunnel: w311 -> [w340 _]
                tunnel: w309 -> [w339 _]
                tunnel: w308 -> [w338 _]
                frame False {
                  n228 = stacked-sequence {
                    seq-local: [w347 _ _ _ _ _] -> [_ w352 _ _ _ _]
                    seq-local: [_ w356 _ _ _ _] -> [_ _ _ w362 _ _]
                    seq-local: [_ _ _ w363 _ _] -> [_ _ _ _ w370 _]
                    seq-local: [_ _ _ _ w368 _] -> [_ _ _ _ _ w375]
                    tunnel: w344 -> [_ _ _ w359 _ w376]
                    tunnel: w343 -> [w348 _ _ _ _ _]
                    tunnel: w342 -> [_ w355 _ _ w369 _]
                    tunnel: w341 -> [w346 _ _ _ _ _]
                    tunnel: w340 -> [_ w350 _ _ _ w377]
                    tunnel: w339 -> [_ _ _ w360 _ w372]
                    tunnel: w338 -> [_ _ _ w361 _ w371]
                    frame #0 {
                      n229 = call-dynamic "Prober_ChuckUpDown.vi"("error in (no error)"=w348, "Direction"=enum16{"up", "down"}."down", "ProbeStationControl in"=w346) -> ("error out"=w347:errorcluster)  [unwired: 6 in, 2 out]
                    }
                    frame #1 {
                      n230 = local write "Status:"("Trimming LCR ..." ("STATUS 1")) -> ()
                      n231 = call-dynamic "Supply_ZeroCheck.vi"("error in (no error)"=w352, "enable/disable"=TRUE, "SupplyControl in"=w350) -> ("error out"=w351:errorcluster)  [unwired: 7 in, 1 out]
                      n232 = call-dynamic "LCR_Init.vi"("error in (no error)"=w351, "LCRControl in"=w355) -> ("error out"=w356:errorcluster)  [unwired: 8 in, 1 out]
                    }
                    frame #2 {
                      n233 = Wait (ms)(milliseconds to wait=u32 1000) -> ()  [unwired: 1 out]
                    }
                    frame #3 {
                      n234 = Wait (ms)(milliseconds to wait=1000) -> ()  [unwired: 1 out]
                      n235 = call-dynamic "MuxCardSwitch.vi"("Single Needle"=w361, "Probe Card Channels"=w360, "error in (no error)"=w362, "Switch to channel"=1, "Switching in"=w359) -> ("error out"=w364:errorcluster, "Switching out"=w358:refnum<class "Switching.lvclass">)  [unwired: 4 in, 1 out]
                      n236 = call-dynamic "MatrixSwitch.vi"("error in (no error)"=w364, "Action"=T5."Striptest LCR", "Switching in"=w358) -> ("error out"=w363:errorcluster)  [unwired: 6 in, 2 out]
                    }
                    frame #4 {
                      n237 = call-dynamic "LCR_TrimOC.vi"("error in (no error)"=w370, "LCRControl in"=w369) -> ("error out"=w368:errorcluster)  [unwired: 8 in, 1 out]
                    }
                    frame #5 {
                      w383 = u16 0 items=["Open", "Close"] ("Switch action")
                      n238 = call-dynamic "Supply_ZeroCheck.vi"("error in (no error)"=w375, "enable/disable"=TRUE, "SupplyControl in"=w377) -> ("error out"=w374:errorcluster)  [unwired: 7 in, 1 out]
                      n239 = call-dynamic "MatrixSwitchSingle.vi"("Switch action"=w383, "error in (no error)"=w374, "Matrix Y"=1, "Matrix X"=3, "Switching in"=w376) -> ("error out"=w379:errorcluster, "Switching out"=w380:refnum<class "Switching.lvclass">)  [unwired: 4 in, 1 out]
                      n240 = call-dynamic "MatrixSwitchSingle.vi"("Switch action"=w383, "error in (no error)"=w379, "Matrix Y"=2, "Matrix X"=4, "Switching in"=w380) -> ("error out"=w378:errorcluster, "Switching out"=w373:refnum<class "Switching.lvclass">)  [unwired: 4 in, 1 out]
                      n241 = call-dynamic "MuxCardSwitch.vi"("Single Needle"=w371, "Probe Card Channels"=w372, "error in (no error)"=w378, "Switch to channel"=-1, "Switching in"=w373) -> ()  [unwired: 4 in, 3 out]
                    }
                  }
                  n242 = local write "Bias On/Off:"(TRUE ("Bias On?")) -> ()
                }
                frame True {
                  n243 = property on="Bias On/Off:" class="Bool (strict)"("Blinking"=w389) -> ()  [unwired: 2 in, 2 out]
                  n244 = local write "Status:"("Compliance exceeded\nRUN ABORTED") -> ()
                }
              }
            }
            frame True {
            }
          }
        }
        frame #3 {
          n245 = property on="Bias On/Off:" class="Bool (strict)"() -> ("Blinking"=w391:bool)  [unwired: 2 in, 2 out]
          n246 = case shown="False" w391 {
            tunnel: w392 -> [w396 _]
            tunnel: w390 -> [w393 _]
            frame False {
              w397 = 0
              n247 = property on="Abort" class="Bool (strict)"("DisabledEnum"=w397) -> ()  [unwired: 2 in, 2 out]
              n248 = property on="Auto ReCheck" class="Bool (strict)"("DisabledEnum"=w397) -> ()  [unwired: 2 in, 2 out]
              n249 = local read "Single Needle"() -> (w395:bool)
              n250 = Or(x=w395, y=w396) -> (x .or. y?=w394:bool)
              n251 = case shown="False" w394 {
                tunnel: [w400 FALSE] -> w398
                tunnel: w393 -> [w399 _]
                frame False {
                  n252 = stacked-sequence {
                    tunnel: [_ w409] -> w400
                    tunnel: w399 -> [_ _]
                    frame #0 {
                      n253 = local write "Status:"("Reference measurement") -> ()
                      n254 = global read "QC_MeasurementSetup.vi" "Striptest Measurement Parameters"() -> (w401:T7)
                      n255 = Unbundle By Name(w401) -> ("Switching"=w402:refnum<class "Switching.lvclass">)
                      n256 = call-dynamic "MatrixSwitch.vi"("Action"=T5."Striptest SMU", "Switching in"=w402) -> ()  [unwired: 7 in, 3 out]
                    }
                    frame #1 {
                      n257 = local read "settling\ndelay [ms]"() -> (w408:i32)
                      n258 = call "CurrentCorrection.vi"("Action"=T6."Reference measurement", "settling\ndelay"=w408) -> ("Compliance exceeded?"=w409:bool, "Current Reference 100V"=→"Current Reference 100V":dbl[], "Current Reference 10V"=→"Current Reference 10V":dbl[])  [unwired: 3 in, 2 out]
                    }
                  }
                }
                frame True {
                }
              }
              n259 = case shown="False" w398 {
                frame False {
                  n260 = local write "Status:"("RUN IN PROGRESS" ("STATUS 1")) -> ()
                }
                frame True {
                  n261 = property on="Bias On/Off:" class="Bool (strict)"("Blinking"=TRUE ("Compliance?")) -> ()  [unwired: 2 in, 2 out]
                  n262 = local write "Status:"("Compliance exceeded\nRUN ABORTED") -> ()
                }
              }
            }
            frame True {
            }
          }
        }
        frame #4 {
          n263 = property on="Bias On/Off:" class="Bool (strict)"() -> ("Blinking"=w416:bool)  [unwired: 2 in, 2 out]
          n264 = case shown="False" w416 {
            tunnel: w417 -> [w427 _]
            tunnel: w415 -> [w426 _]
            tunnel: w414 -> [w425 _]
            frame False {
              n265 = Array Size(array=w427) -> (size(s)=w428:i32)
              n266 = local read "Temperature Progression"() -> (w419:T3)
              n267 = local read "probe points per region"() -> (w420:i32[])
              n268 = local read "max scale array"() -> (w423:i32[])
              n269 = local read "min scale array"() -> (w422:i32[])
              n270 = for {
                N: w428 -> [_]
                tunnel: w427 -> [w441] mode=indexing
                tunnel: w426 -> [w440] mode=indexing
                tunnel: w425 -> [w439]
                shift-right: [w433] -> _
                shift-left: 0 -> [w438]
                tunnel: w423 -> [w436] mode=indexing
                tunnel: w422 -> [w437] mode=indexing
                shift-right: [w432] -> _
                shift-left: 0 -> [w434]
                tunnel: w420 -> [w431] mode=indexing
                shift-right: [w429] -> w418
                shift-left: w419 -> [w430]
                i -> [w435]
                n271 = case shown="True" w441 {
                  tunnel: w440 -> [_ w457]
                  tunnel: w439 -> [_ _]
                  tunnel: w438 -> [w443 w458]
                  tunnel: w437 -> [_ w453]
                  tunnel: w436 -> [_ w450]
                  tunnel: w435 -> [_ w455]
                  tunnel: w434 -> [w445 w452]
                  tunnel: [w442 w451] -> w433
                  tunnel: [w445 w449] -> w432
                  tunnel: w431 -> [_ w448]
                  tunnel: w430 -> [w444 w447]
                  tunnel: [w444 w446] -> w429
                  frame False {
                    n272 = Increment(x=w443) -> (x+1=w442:i32)
                  }
                  frame True {
                    n273 = local write "Show:"(w458) -> ()
                    n274 = Unbundle By Name(w457) -> ("Region"=→"Probing Region:":string, "ProbePoints"=w454:T13)
                    n275 = Increment(x=w458) -> (x+1=w451:i32)
                    n276 = while {
                      tunnel: w455 -> [w459]
                      tunnel: w454 -> [w479]
                      shift-right: [w472] -> _
                      shift-left: w453 -> [w461]
                      shift-right: [w473] -> w449
                      shift-left: w452 -> [w474]
                      tunnel: w450 -> [w471]
                      tunnel: w448 -> [_]
                      shift-right: [w469] -> w446
                      shift-left: w447 -> [w470]
                      i -> [w475]
                      stop <- w478 stop-if-true
                      n277 = Index Array(array=w479, index=w461) -> (element=w480:T14)
                      n278 = Equal To 0?(x=w474) -> (x = 0?=w481:bool)
                      n279 = Equal?(x=w461, y=w471) -> (x = y?=w460:bool)
                      n280 = case shown="True" w481 {
                        frame False {
                        }
                        frame True {
                          n281 = local read "Probe Card Channels"() -> (w1029:i32)
                          n282 = local read "total strip number"() -> (w1030:u32)
                          n283 = Divide(x=w1030, y=w1029) -> (x/y=w1028:dbl)
                          n284 = To Long Integer(number=w1028) -> (32bit integer=w1027:i32)
                          n285 = call "RunTime.vi"("no. measurements"=w1027, "Flag"=1) -> ()  [unwired: 2 in, 4 out]
                        }
                      }
                      n286 = case shown="True" w460 {
                        tunnel: w459 -> [_ w482]
                        frame False {
                        }
                        frame True {
                          n287 = stacked-sequence {
                            tunnel: w482 -> [_ w485 w491]
                            frame #0 {
                              n288 = Wait (ms)(milliseconds to wait=100) -> ()  [unwired: 1 out]
                            }
                            frame #1 {
                              n289 = Increment(x=w485) -> (x+1=w488:i32)
                              n290 = Multiply(x=w488, y=111) -> (x*y=w486:i32)
                              n291 = call "SaveJPEG.vi"("Picture No."=w486, "Test"="Striptest") -> ()  [unwired: 1 in, 2 out]
                            }
                            frame #2 {
                              n292 = local read "probe points per region"() -> (w495:i32[])
                              n293 = Index Array(array=w495, index=w491) -> (element=w492:i32)
                              n294 = local read "Probing Region:"() -> (w490:string)
                              n295 = call "SaveStriptestRecoveryFiles.vi"("Arrays format"="%016.6f", "Array Titles"="ProbeplanIndex Current PinholeFlag Capacitance Resistance", "Strip Segment"=w490, "no. of arrays"=5, "Actual array lengths"=w492, "Region #"=w491) -> ()  [unwired: 2 out]
                            }
                          }
                        }
                      }
                      n296 = Unbundle By Name(w480) -> ("CardViable?"=w466:bool)
                      n297 = property on="Bias On/Off:" class="Bool (strict)"() -> ("Blinking"=w476:bool)  [unwired: 2 in, 2 out]
                      n298 = property on="Bias On/Off:" class="Bool (strict)"() -> ("Blinking"=w468:bool)  [unwired: 2 in, 2 out]
                      n299 = local read "Abort"() -> (w464:bool)
                      n300 = Not(x=w468) -> (.not. x?=w467:bool)
                      n301 = Not(x=w464) -> (.not. x?=w463:bool)
                      n302 = Compound Arithmetic op=AND(w466, w467, w463) -> (w465:bool)
                      n303 = Build Array(w476, "Abort", w460) -> (w477:bool[])
                      n304 = Or Array Elements(Boolean array=w477) -> (logical OR=w478:bool)
                      n305 = case shown="True" w465 {
                        tunnel: w459 -> [_ w513]
                        tunnel: w479 -> [_ w512]
                        tunnel: w461 -> [w496 w507]
                        tunnel: w475 -> [_ w511]
                        tunnel: w474 -> [w499 w510]
                        tunnel: [w499 w509] -> w473
                        tunnel: [w497 w508] -> w472
                        tunnel: w470 -> [w498 w506]
                        tunnel: [w498 w505] -> w469
                        frame False {
                          n306 = Increment(x=w496) -> (x+1=w497:i32)
                        }
                        frame True {
                          n307 = global read "QC_MeasurementSetup.vi" "Striptest Measurement Parameters"() -> (w503:T7)
                          n308 = Unbundle By Name(w503) -> ("ProbeStation"=w502:refnum<class "ProbeStationControl.lvclass">, "Switching"=w504:refnum<class "Switching.lvclass">, "Temperature Readout"=w500:enum16{"Read Arduino", "Enter manually"}, "Arduino"=w501:refnum<class "ArduinoControl.lvclass">)
                          n309 = stacked-sequence {
                            tunnel: w513 -> [w527 w808 w898 w987 _]
                            tunnel: w512 -> [w516 _ _ _ _]
                            tunnel: w507 -> [w515 _ _ _ w1014]
                            tunnel: w510 -> [_ _ _ _ w1025]
                            tunnel: w511 -> [_ w807 w897 w986 w1012]
                            tunnel: [_ _ _ _ w1015] -> w509
                            tunnel: [_ _ _ _ w1024] -> w508
                            tunnel: w506 -> [_ w802 _ _ _]
                            tunnel: [_ w801 _ _ _] -> w505
                            tunnel: w504 -> [_ w805 w895 _ _]
                            tunnel: w502 -> [w514 _ _ _ _]
                            tunnel: w501 -> [_ w804 _ _ _]
                            tunnel: w500 -> [_ w803 _ _ _]
                            frame #0 {
                              w526 = u32 4 items=["Reset", "Read Array", "Read Element", "Write Element", "Write Array"] ("Action")
                              # "If probepoint label defined as Strip or Channel, use\nthat as the channel number in the data array."
                              n310 = local write "disabled channels"(i32[] []) -> ()
                              n311 = Index Array(array=w516, index=w515) -> (element=w534:T14)
                              n312 = Unbundle(w534) -> ("Label"=w530:string)  [unwired: 3 out]
                              "Probe Point:" <- w530
                              n313 = local read "Simulation?"() -> (w520:bool)
                              n314 = local read "Abort"() -> (w522:bool)
                              n315 = Format Into String(format string="Moving to %s", w530) -> (resulting string=w533:string)  [unwired: 2 in, 1 out]
                              n316 = local write "Status:"(w533) -> ()
                              n317 = local read "Probe Card Channels"() -> (w523:i32)
                              n318 = Or(x=w522, y=w520) -> (x .or. y?=w521:bool)
                              n319 = case shown="False" w521 {
                                tunnel: w527 -> [w793 _]
                                tunnel: w515 -> [w794 _]
                                tunnel: w523 -> [w795 _]
                                tunnel: w514 -> [w791 _]
                                frame False {
                                # "Move to Strip"
                                n320 = local read "Single Needle"() -> (w797:bool)
                                n321 = call "MoveToStrip.vi"("Single Needle"=w797, "Strip No."=w794, "Region"=w793, "ProbeStationControl in"=w791) -> ("Z [µm]"=w792:i32)  [unwired: 5 in, 2 out]
                                n322 = local read "Z profile"() -> (w800:i32[][])
                                n323 = Initialize Array(w792, w795, 1) -> (w798:i32[][])
                                n324 = Replace Array Subset(array=w800, new element=w798, index (row)=w794, index (col)=w793) -> (w799:i32[][])
                                n325 = local write "Z profile"(w799) -> ()
                                }
                                frame True {
                                }
                              }
                              n326 = xnode "Match Regular Expression"("input string"=w530, "regular expression"="(Strip|Channel)\\s+(\\d+)", "ignore case? (F)"=TRUE) -> ("submatch 2"=w519:string)  [unwired: 3 in, 6 out]
                              n327 = Empty String/Path?(string/path=w519) -> (empty?=w518:bool)
                              n328 = Not(x=w518) -> (.not. x?=w517:bool)
                              n329 = case shown="True" w517 {
                                tunnel: [w536 w546] -> w528
                                tunnel: w515 -> [w538 w544]
                                tunnel: w523 -> [w537 w545]
                                tunnel: w516 -> [_ w543]
                                frame False {
                                n330 = for {
                                N: w537 -> [_]
                                tunnel: w538 -> [w541]
                                tunnel: [w539] -> w536 mode=indexing
                                i -> [w542]
                                # "Actually use the probepoint\nindex"
                                n331 = Add(x=w541, y=w542) -> (x+y=w540:i32)
                                n332 = Increment(x=w540) -> (x+1=w539:i32)
                                }
                                }
                                frame True {
                                n333 = for {
                                N: w545 -> [_]
                                tunnel: [w555] -> w546 mode=indexing
                                tunnel: w544 -> [w552]
                                tunnel: w543 -> [w550]
                                i -> [w553]
                                n334 = Add(x=w552, y=w553) -> (x+y=w551:i32)
                                n335 = Index Array(array=w550, index=w551) -> (element=w549:T14)
                                n336 = Unbundle By Name(w549) -> ("Label"=w548:string)
                                n337 = xnode "Match Regular Expression"("input string"=w548, "regular expression"="(Strip|Channel)\\s+(\\d+)") -> ("submatch 2"=w547:string)  [unwired: 4 in, 6 out]
                                n338 = Scan From String(format string="%d", input string=w547) -> (output 1=w555:i32)  [unwired: 3 in, 3 out]
                                }
                                }
                              }
                              n339 = To Double Precision Float(number=w528) -> (double precision float=w524:dbl[])
                              n340 = call "MultiRegionData.vi"("Action"=w526, "Array No."=0 ("Array Size / Index"), "Array Size / Index"=w515, "Array IN"=w524, "Region index"=w527) -> ()  [unwired: 1 in, 2 out]
                            }
                            frame #1 {
                              # "Pinholes"
                              n341 = local read "Simulation?"() -> (w806:bool)
                              n342 = stacked-sequence {
                                tunnel: w806 -> [w824 w845]
                                tunnel: w808 -> [_ w847]
                                tunnel: w807 -> [_ w846]
                                tunnel: w805 -> [w823 _]
                                tunnel: w804 -> [w821 _]
                                tunnel: w803 -> [w822 _]
                                tunnel: w802 -> [w815 _]
                                tunnel: [w813 _] -> w801
                                frame #0 {
                                n343 = Unbundle By Name(w815) -> ("Time Array"=w817:string[], "Temperature Array [°C]"=w812:dbl[], "Humidity Array [RH %]"=w811:dbl[])
                                n344 = case shown="\"Read Arduino\", Default" w822 {
                                tunnel: w821 -> [w832 _]
                                tunnel: [w831 _] -> w820
                                tunnel: w812 -> [w827 w836]
                                tunnel: w811 -> [w828 w838]
                                tunnel: [w826 w835] -> w810
                                tunnel: [w825 w834] -> w809
                                frame "Read Arduino", Default {
                                n345 = call "ArduinoRead.vi"("Arduino function"=enum16{"T/RH", "Interlock", "Edgesense"}."T/RH", "ArduinoControl in"=w832) -> ("error out"=w831:errorcluster, "rel. Humidity [%]"=w829:dbl, "Temperature [°C]"=w830:dbl)  [unwired: 4 in, 3 out]
                                n346 = Build Array (concatenate)(w827, w830) -> (w826:dbl[])
                                n347 = Build Array (concatenate)(w828, w829) -> (w825:dbl[])
                                }
                                frame "Enter manually" {
                                n348 = Index Array(array=w836, index=0) -> (element=w837:dbl)
                                n349 = Index Array(array=w838, index=0) -> (element=w839:dbl)
                                n350 = Build Array (concatenate)(w836, w837) -> (w835:dbl[])
                                n351 = Build Array (concatenate)(w838, w839) -> (w834:dbl[])
                                }
                                }
                                n352 = call "RunTime.vi"("Probing done - new estimation"=FALSE, "Flag"=0) -> ("Time so far"=w816:string)  [unwired: 2 in, 3 out]
                                n353 = Build Array (concatenate)(w817, w816) -> (w814:string[])
                                n354 = case shown="False" w824 {
                                tunnel: w823 -> [w844 _]
                                tunnel: w820 -> [w843 _]
                                frame False {
                                n355 = call-dynamic "MatrixSwitch.vi"("error in (no error)"=w843, "Action"=T5."Striptest SMU", "Switching in"=w844) -> ()  [unwired: 6 in, 3 out]
                                }
                                frame True {
                                }
                                }
                                n356 = Bundle By Name(cluster=w815, "Time Array"=w814, "Temperature Array [°C]"=w810, "Humidity Array [RH %]"=w809) -> (w813:T3)
                                }
                                frame #1 {
                                n357 = local read "Abort"() -> (w848:bool)
                                n358 = case shown="False" w848 {
                                tunnel: w847 -> [w858 _]
                                tunnel: w846 -> [w857 _]
                                tunnel: w845 -> [w849 _]
                                frame False {
                                w854 = u32 4 items=["Reset", "Read Array", "Read Element", "Write Element", "Write Array"] ("Action")
                                w855 = u32 4 items=["Reset", "Read Array", "Read Element", "Write Element", "Write Array"] ("Action")
                                n359 = case shown="True" w849 {
                                tunnel: [w870 w883] -> w850
                                tunnel: [w867 w882] -> w856
                                frame False {
                                n360 = local read "Thresholds:"() -> (w869:T2)
                                n361 = Unbundle By Name(w869) -> ("Current [nA]"=w868:dbl)
                                n362 = case shown="False" "Rolling\nCurrent Readout" {
                                tunnel: [w875 w877] -> w870
                                tunnel: w868 -> [w871 w880]
                                tunnel: [w874 w879] -> w867
                                tunnel: [w873 w878] -> w866
                                tunnel: "settling\ndelay [ms]" -> [w872 w876]
                                frame False {
                                n363 = call "Pinholes.vi"("Current Threshold [nA]"=w871, "settling\ndelay"=w872) -> ("excluded channels"=w873:i32[], "Current [nA]"=w875:dbl[], "Flag"=w874:i32[])  [unwired: 3 in]
                                }
                                frame True {
                                n364 = call "PinholesRolling.vi"("Current Threshold [nA]"=w880, "settling\ndelay"=w876) -> ("excluded channels"=w878:i32[], "Current [nA]"=w877:dbl[], "Flag"=w879:i32[])  [unwired: 3 in]
                                }
                                }
                                "disabled channels" <- w866
                                }
                                frame True {
                                n365 = local read "Probe Card Channels"() -> (w881:i32)
                                n366 = for {
                                N: w881 -> [_]
                                tunnel: [w885] -> w883 mode=indexing
                                tunnel: [w884] -> w882 mode=indexing
                                # "Simulate"
                                n367 = Random Number (0-1)() -> (number: 0 to 1=w888:dbl)
                                n368 = Greater?(x=w888, y=0.95) -> (0:w889:bool)
                                n369 = case shown="False" w889 {
                                tunnel: [w893 5000.0] -> w885
                                tunnel: w888 -> [w893 _]
                                frame False {
                                }
                                frame True {
                                }
                                }
                                n370 = Greater?(x=w885, y=50.0) -> (0:w886:bool)
                                n371 = case shown="False" w886 {
                                tunnel: [0 1] -> w884
                                frame False {
                                }
                                frame True {
                                }
                                }
                                }
                                }
                                }
                                n372 = Get Date/Time String(want seconds? (F)=TRUE) -> (time string=→"Last Probe at:":string)  [unwired: 2 in, 1 out]
                                n373 = local write "Status:"("Measuring Ipinhole") -> ()
                                n374 = To Double Precision Float(number=w856) -> (double precision float=w853:dbl[])
                                n375 = Index Array(array=w850, index=0) -> (element=→"Current [nA]:":dbl)
                                n376 = call "MultiRegionData.vi"("Action"=w854, "Array No."=1, "Array Size / Index"=w857, "Array IN"=w850, "Region index"=w858) -> ()  [unwired: 1 in, 2 out]
                                n377 = call "MultiRegionData.vi"("Action"=w855, "Array No."=2, "Array Size / Index"=w857, "Array IN"=w853, "Region index"=w858) -> ()  [unwired: 1 in, 2 out]
                                }
                                frame True {
                                }
                                }
                                }
                              }
                            }
                            frame #2 {
                              # "Capacitance and Resistance"
                              n378 = local read "Simulation?"() -> (w896:bool)
                              n379 = stacked-sequence {
                                seq-local: [_ _ w910 _] -> [_ _ _ w971]
                                tunnel: w898 -> [_ _ w920 _]
                                tunnel: w897 -> [_ _ w919 _]
                                tunnel: w896 -> [w900 w904 w909 w970]
                                tunnel: w895 -> [w899 w903 w908 w969]
                                frame #0 {
                                n380 = case shown="False" w900 {
                                tunnel: w899 -> [w901 _]
                                frame False {
                                n381 = call-dynamic "MatrixSwitch.vi"("Action"=T5."Ground", "Switching in"=w901) -> ()  [unwired: 7 in, 3 out]
                                }
                                frame True {
                                }
                                }
                                }
                                frame #1 {
                                n382 = case shown="False" w904 {
                                tunnel: w903 -> [w906 _]
                                frame False {
                                n383 = call-dynamic "MatrixSwitch.vi"("Action"=T5."Striptest LCR", "Switching in"=w906) -> ()  [unwired: 7 in, 3 out]
                                }
                                frame True {
                                }
                                }
                                n384 = local write "Status:"("Measuring capacitance..." ("STATUS 1")) -> ()
                                }
                                frame #2 {
                                w913 = 0
                                w917 = u32 4 items=["Reset", "Read Array", "Read Element", "Write Element", "Write Array"] ("Action")
                                w918 = u32 4 items=["Reset", "Read Array", "Read Element", "Write Element", "Write Array"] ("Action")
                                n385 = local read "Probe Card Channels"() -> (w910:i32)
                                n386 = local read "disabled channels"() -> (w912:i32[])
                                n387 = for {
                                N: w910 -> [_]
                                tunnel: [w929] -> w911 mode=indexing
                                tunnel: [w928] -> w914 mode=indexing
                                tunnel: w912 -> [w925]
                                tunnel: w910 -> [w927]
                                tunnel: w909 -> [w924]
                                tunnel: w908 -> [w923]
                                i -> [w926]
                                n388 = case shown="False" w924 {
                                tunnel: [w938 w960] -> w929
                                tunnel: [w937 w959] -> w928
                                tunnel: w927 -> [w934 _]
                                tunnel: w926 -> [w932 _]
                                tunnel: w925 -> [w933 _]
                                tunnel: w923 -> [w930 _]
                                frame False {
                                n389 = Increment(x=w932) -> (x+1=w931:i32)
                                n390 = Search 1D Array(1D array=w933, element=w931) -> (index of element=w936:i32)  [unwired: 1 in]
                                n391 = Less Than 0?(x=w936) -> (x < 0?=w935:bool)
                                n392 = case shown="True" w935 {
                                tunnel: [w941 w947] -> w938
                                tunnel: [w939 w946] -> w937
                                tunnel: w934 -> [_ w945]
                                tunnel: w931 -> [_ w944]
                                tunnel: w933 -> [_ w943]
                                tunnel: w930 -> [_ w942]
                                frame False {
                                w941 = -1.0
                                n393 = Divide(x=w941, y=1000000.0) -> (x/y=w939:dbl)
                                }
                                frame True {
                                n394 = stacked-sequence {
                                tunnel: w945 -> [w950 _ _]
                                tunnel: w944 -> [w952 _ _]
                                tunnel: w943 -> [w951 _ _]
                                tunnel: [_ _ w958] -> w947
                                tunnel: [_ _ w957] -> w946
                                tunnel: w942 -> [w949 _ _]
                                frame #0 {
                                n395 = local read "Single Needle"() -> (w948:bool)
                                n396 = call-dynamic "MuxCardSwitch.vi"("Single Needle"=w948, "Probe Card Channels"=w950, "disabled channels"=w951, "Switch to channel"=w952, "Switching in"=w949) -> ()  [unwired: 4 in, 3 out]
                                }
                                frame #1 {
                                n397 = local read "settling\ndelay [ms]"() -> (w953:i32)
                                n398 = Wait (ms)(milliseconds to wait=w953) -> ()  [unwired: 1 out]
                                }
                                frame #2 {
                                n399 = global read "QC_MeasurementSetup.vi" "Striptest Measurement Parameters"() -> (w956:T7)
                                n400 = Unbundle By Name(w956) -> ("LCR"=w955:refnum<class "LCRControl.lvclass">, "AC frequency [Hz]"=w954:i32)
                                n401 = call-dynamic "LCR_Readout.vi"("Frequency in Hz"=w954, "LCRControl in"=w955) -> ("Resistance in Ohm"=w957:dbl, "Capacitance in pF"=w958:dbl)  [unwired: 6 in, 2 out]
                                }
                                }
                                }
                                }
                                }
                                frame True {
                                n402 = Random Number (0-1)() -> (number: 0 to 1=w964:dbl)
                                n403 = Random Number (0-1)() -> (number: 0 to 1=w968:dbl)
                                n404 = Multiply(x=w968, y=18.0) -> (x*y=w966:dbl)
                                n405 = Multiply(x=w964, y=0.6) -> (x*y=w961:dbl)
                                n406 = Add(x=w966, y=64.0) -> (x+y=w960:dbl)
                                n407 = Add(x=1.5 ("Resistance"), y=w961) -> (x+y=w959:dbl)
                                }
                                }
                                }
                                n408 = Index Array(array=w914, index=w913) -> (element=→"Reistance [MW]:":dbl)
                                n409 = Index Array(array=w911, index=w913) -> (element=→"Capacitance [pF]:":dbl)
                                n410 = call "MultiRegionData.vi"("Action"=w918, "Array No."=3, "Array Size / Index"=w919, "Array IN"=w911, "Region index"=w920) -> ()  [unwired: 1 in, 2 out]
                                n411 = call "MultiRegionData.vi"("Action"=w917, "Array No."=4, "Array Size / Index"=w919, "Array IN"=w914, "Region index"=w920) -> ()  [unwired: 1 in, 2 out]
                                }
                                frame #3 {
                                n412 = case shown="False" w970 {
                                tunnel: w971 -> [w974 _]
                                tunnel: w969 -> [w972 _]
                                frame False {
                                n413 = local read "Single Needle"() -> (w973:bool)
                                n414 = call-dynamic "MuxCardSwitch.vi"("Single Needle"=w973, "Probe Card Channels"=w974, "Switch to channel"=-1, "Switching in"=w972) -> ()  [unwired: 5 in, 3 out]
                                }
                                frame True {
                                }
                                }
                                }
                              }
                            }
                            frame #3 {
                              # "If selected region is CURRENT region being probed,\nuse number probed so far\notherwise total number of probepoints in this region"
                              n415 = local read "Region Indices"() -> (w989:i32[])
                              n416 = Index Array(array=w989, index="Show:") -> (element=w985:i32)
                              n417 = Equal?(x=w985, y=w987) -> (x = y?=w988:bool)
                              n418 = case shown="True" w988 {
                                tunnel: w986 -> [_ w1002]
                                tunnel: [w998 w1001] -> w984
                                tunnel: w985 -> [w997 _]
                                frame False {
                                n419 = local read "probe points per region"() -> (w999:i32[])
                                n420 = Index Array(array=w999, index=w997) -> (element=w998:i32)
                                }
                                frame True {
                                n421 = local read "Probe Card Channels"() -> (w1000:i32)
                                n422 = Add(x=w1000, y=w1002) -> (x+y=w1001:i32)
                                }
                              }
                              n423 = local read "max scale array"() -> (w981:i32[])
                              n424 = local read "min scale array"() -> (w983:i32[])
                              n425 = local read "Thresholds:"() -> (w996:T2)
                              n426 = Index Array(array=w981, index="Show:") -> (element=w978:i32)
                              n427 = Index Array(array=w983, index="Show:") -> (element=w980:i32)
                              n428 = call "DisplayStriptestData.vi"("min scale array"=w983, "max scale array"=w981, "# probed"=w984, "Display Stats?"="Display Stats", "Thresholds"=w996, "Region"=w985) -> ("Defects"=w991:i32[][], "Resistance [MW]"=→"Resistance [MW]":cluster{u32, i32, "Array OUT":dbl[]}, "Capacitance [pF]"=→"Capacitance [pF]":cluster{u32, i32, "Array OUT":dbl[]}, "Current [nA]"=→"Current [nA]":cluster{u32, i32, "Array OUT":dbl[]}, "Strip Quality Data"=w992:T15)
                              n429 = case shown="True" "Display Stats" {
                                tunnel: w992 -> [_ w1008]
                                tunnel: w991 -> [_ w1007]
                                frame False {
                                }
                                frame True {
                                n430 = Unbundle By Name(w1008) -> ("pass Rate in %"=→"% OK:":dbl, "Bad channel list"=→"Bad Strip List":i32[], "No of bad strips"=w1006:i32, "Number of defects per category"=→"defect type array":i32[])
                                n431 = local write "# total defects:"(w1006) -> ()
                                "Defects" <- w1007
                                }
                              }
                              n432 = Increment(x=w978) -> (x+1=w977:i32)
                              n433 = Increment(x=w980) -> (x+1=w979:i32)
                              n434 = property on="Capacitance [pF]" class="WFGraph (strict)"("XScale.Maximum"=w977) -> ()  [unwired: 2 in, 2 out]
                              n435 = property on="Resistance [MW]" class="WFGraph (strict)"("XScale.Maximum"=w977) -> ()  [unwired: 2 in, 2 out]
                              n436 = property on="Current [nA]" class="WFGraph (strict)"("XScale.Maximum"=w977) -> ()  [unwired: 2 in, 2 out]
                              n437 = property on="Capacitance [pF]" class="WFGraph (strict)"("XScale.Minimum"=w979) -> ()  [unwired: 2 in, 2 out]
                              n438 = property on="Resistance [MW]" class="WFGraph (strict)"("XScale.Minimum"=w979) -> ()  [unwired: 2 in, 2 out]
                              n439 = property on="Current [nA]" class="WFGraph (strict)"("XScale.Minimum"=w979) -> ()  [unwired: 2 in, 2 out]
                              n440 = property on="Defects" class="IntGraph (strict)"("XScale.Minimum"=w979) -> ()  [unwired: 2 in, 2 out]
                              n441 = Increment(x=w977) -> (x+1=w976:i32)
                              n442 = property on="Defects" class="IntGraph (strict)"("XScale.Maximum"=w976) -> ()  [unwired: 2 in, 2 out]
                            }
                            frame #4 {
                              # "save image if required"
                              n443 = call "RunTime.vi"("Probing done - new estimation"=TRUE, "Flag"=0) -> ("Estimated Completion Time"=w1021:string, "Time so far"=→"Run Duration:":string)  [unwired: 2 in, 2 out]
                              n444 = Greater Or Equal?(x=w1012, y=20) -> (x >= y?=w1018:bool)
                              n445 = Scan From String(format string="%s %s", input string=w1021) -> (output 2=→"Estimated Completion:":string)  [unwired: 5 in, 3 out]
                              n446 = case shown="True" w1018 {
                                selector: w1018 -> [_ w1026]
                                frame False {
                                }
                                frame True {
                                # "Start calculating stats after 20 strips"
                                n447 = local write "Display Stats"(w1026) -> ()
                                }
                              }
                              n448 = local read "Probe Card Channels"() -> (w1013:i32)
                              n449 = Quotient & Remainder(x=w1012, y=w1013) -> (floor(x/y)=w1011:i32)  [unwired: 1 out]
                              n450 = Add(x=w1013, y=w1025) -> (x+y=w1015:i32)
                              n451 = Increment(x=w1011) -> (x+1=w1010:i32)
                              n452 = local write "# probed"(w1015) -> ()
                              n453 = call "SaveJPEG.vi"("Picture No."=w1010, "Test"="Striptest") -> ()  [unwired: 1 in, 2 out]
                              n454 = Increment(x=w1014) -> (x+1=w1024:i32)
                            }
                          }
                        }
                      }
                    }
                  }
                }
              }
              n455 = local write "Temperature Progression"(w418) -> ()
            }
            frame True {
            }
          }
        }
        frame #5 {
          # "Ramp down volts now"
          n456 = case shown="False" w1033 {
            tunnel: w1032 -> [w1054 _]
            frame False {
              w1059 = "0"
              n457 = property on="Abort" class="Bool (strict)"("DisabledEnum"=2) -> ()  [unwired: 2 in, 2 out]
              n458 = local read "# probed"() -> (w1052:i32)
              n459 = call-dynamic "Prober_ChuckUpDown.vi"("Direction"=enum16{"up", "down"}."down", "ProbeStationControl in"=w1054) -> ("error out"=w1056:errorcluster, "ProbeStationControl out"=w1055:refnum<class "ProbeStationControl.lvclass">)  [unwired: 7 in, 1 out]
              n460 = call "SaveJPEG.vi"("Picture No."=w1052, "Test"="Striptest") -> ()  [unwired: 1 in, 2 out]
              n461 = call-dynamic "Prober_MoveToXYZTheta.vi"("Theta location [mdeg]"="none", "ProbeStationControl in"=w1055, "error in (no error)"=w1056, "Z location [µm]"="down", "Y location [µm]"=w1059, "X location [µm]"=w1059) -> ()  [unwired: 3 in, 3 out]
            }
            frame True {
            }
          }
          n462 = local read "Abort"() -> (w1045:bool)
          n463 = property on="Bias On/Off:" class="Bool (strict)"() -> ("Blinking"=w1044:bool)  [unwired: 2 in, 2 out]
          n464 = Not Or(1:w1045, 2:w1044) -> (0:w1043:bool)
          n465 = Build Array(w1043, w1044, w1045) -> (w1046:bool[])
          n466 = Search 1D Array(1D array=w1046, element=TRUE) -> (index of element=w1048:i32)  [unwired: 1 in]
          n467 = Increment(x=w1048) -> (x+1=w1034:i32)
          n468 = Pick Line(multi-line string=" null\n Run ended normally.\n Compliance exceeded. \n Run aborted early.", line index=w1034) -> (output string=w1035:string)  [unwired: 1 in]
          n469 = global read "QC_RunInformation.vi" "Run info"() -> (w1037:T8)
          n470 = Bundle By Name(cluster=w1037, "End of Run comment:"=w1035) -> (w1036:T8)
          n471 = global write "QC_RunInformation.vi" "Run info"(w1036) -> ()
          n472 = Concatenate Strings(" End of Run.", "\r\n", w1035) -> (w1038:string)
          n473 = Concatenate Strings(w1035, "\r\n", "RAMPING DOWN VOLTS") -> (w1041:string)
          n474 = stacked-sequence {
            tunnel: w1041 -> [w1061 _ _ _]
            tunnel: w1038 -> [_ _ w1065 _]
            frame #0 {
              n475 = local write "Status:"(w1061) -> ()
            }
            frame #1 {
              n476 = local read "Simulation?"() -> (w1062:bool)
              n477 = case shown="False" w1062 {
                frame False {
                  n478 = global read "QC_MeasurementSetup.vi" "Striptest Measurement Parameters"() -> (w1064:T7)
                  n479 = Unbundle By Name(w1064) -> ("SMU"=w1063:refnum<class "SupplyControl.lvclass">)
                  n480 = call-dynamic "Supply_Stby.vi"("SupplyControl in"=w1063) -> ()  [unwired: 9 in, 2 out]
                }
                frame True {
                }
              }
            }
            frame #2 {
              n481 = local write "Status:"(w1065) -> ()
            }
            frame #3 {
              w1068 = 0
              n482 = property on="Save Data" class="Bool (strict)"("DisabledEnum"=w1068) -> ()  [unwired: 2 in, 2 out]
              n483 = property on="Quit w/o saving" class="Bool (strict)"("DisabledEnum"=w1068) -> ()  [unwired: 2 in, 2 out]
              n484 = property on="ReCheck" class="Bool"("DisabledEnum"=w1068) -> ()  [unwired: 2 in, 2 out]
              n485 = property on="Auto ReCheck" class="Bool (strict)"("DisabledEnum"=1) -> ()  [unwired: 2 in, 2 out]
              n486 = local write "Status:"("Run finished. \nSave data?" ("STATUS 1")) -> ()
            }
          }
        }
        frame #6 {
          w1079 = ""
          n487 = stacked-sequence {
            tunnel: [w1101 _ _ _] -> w1097
            tunnel: [w1100 _ _ _] -> w1096
            tunnel: w1090 -> [_ w1204 w1219 _]
            tunnel: w1089 -> [w1099 _ _ _]
            frame #0 {
              # "Loop and await decision on whether to save or junk data"
              n488 = local read "Show:"() -> (w1102:u16)
              n489 = while {
                shift-right: [w1110] -> _
                shift-left: w1102 -> [w1111]
                tunnel: ["Save Data"] -> w1100
                tunnel: ["Quit w/o saving"] -> w1101
                tunnel: w1099 -> [w1103]
                stop <- w1114 stop-if-true
                # "display data if selected region changes"
                n490 = Wait (ms)(milliseconds to wait=u32 200) -> ()  [unwired: 1 out]
                n491 = local read "Show:"() -> (w1112:u16)
                n492 = Not Equal?(x=w1112, y=w1111) -> (x != y?=w1113:bool)
                n493 = Or(x="ReCheck", y="Auto ReCheck") -> (x .or. y?=w1105:bool)
                n494 = case shown="True" w1105 {
                  tunnel: "Auto ReCheck" -> [_ w1116]
                  tunnel: w1103 -> [_ w1115]
                  frame False {
                  }
                  frame True {
                    n495 = case shown="True" w1116 {
                      tunnel: w1115 -> [_ w1146]
                      frame False {
                        n496 = local read "probe points per region"() -> (w1123:i32[])
                        n497 = local read "Region Indices"() -> (w1124:i32[])
                        n498 = local read "Show:"() -> (w1122:u16)
                        n499 = Index Array(array=w1124, index=w1122) -> (element=w1121:i32)
                        n500 = Index Array(array=w1123, index=w1122) -> (element=w1120:i32)
                        n501 = flat-sequence {
                          tunnel: w1121 -> [w1125]
                          tunnel: w1120 -> [w1129]
                          tunnel: [w1125] -> w1119
                          tunnel: [w1129] -> w1118
                          tunnel: [w1128] -> w1117
                          tunnel: w1119 -> [w1145]
                          tunnel: w1118 -> [w1142]
                          tunnel: w1117 -> [w1131]
                          frame #0 {
                            n502 = local read "Probe Card Channels"() -> (w1126:i32)
                            n503 = local read "Auto ReCheck"() -> (w1127:bool)
                            n504 = local read "Thresholds:"() -> (w1130:T2)
                            n505 = call "ReCheckStrips.vi"("Probe Card Channels"=w1126, "Auto Re-Check"=w1127, "Thresholds"=w1130, "region in"=w1125, "Number of strips probed"=w1129) -> ("Thresholds copy"=w1128:T16)  [unwired: 6 in]
                            n506 = local write "Thresholds:"(w1128) -> ()
                          }
                          frame #1 {
                            n507 = local read "max scale array"() -> (w1144:i32[])
                            n508 = local read "min scale array"() -> (w1143:i32[])
                            n509 = call "DisplayStriptestData.vi"("min scale array"=w1143, "max scale array"=w1144, "# probed"=w1142, "Display Stats?"=TRUE, "Thresholds"=w1131, "Region"=w1145) -> ("Defects"=w1137:i32[][], "Resistance [MW]"=w1138:cluster{u32, i32, "Array OUT":dbl[]}, "Capacitance [pF]"=w1140:cluster{u32, i32, "Array OUT":dbl[]}, "Current [nA]"=w1139:cluster{u32, i32, "Array OUT":dbl[]}, "Strip Quality Data"=w1136:T15)
                            n510 = Unbundle By Name(w1136) -> ("pass Rate in %"=w1135:dbl, "Bad channel list"=w1134:i32[], "No of bad strips"=w1133:i32, "Defect description list"=w1132:i32[])
                            n511 = local write "Current [nA]"(w1139) -> ()
                            n512 = local write "Capacitance [pF]"(w1140) -> ()
                            n513 = local write "Resistance [MW]"(w1138) -> ()
                            n514 = local write "Defects"(w1137) -> ()
                            n515 = local write "% OK:"(w1135) -> ()
                            n516 = local write "Bad Strip List"(w1134) -> ()
                            n517 = local write "# total defects:"(w1133) -> ()
                            n518 = local write "defect type array"(w1132) -> ()
                          }
                        }
                      }
                      frame True {
                        n519 = flat-sequence {
                          tunnel: w1146 -> [w1147]
                          frame #0 {
                            n520 = local read "Region Indices"() -> (w1148:i32[])
                            n521 = Array Size(array=w1148) -> (size(s)=w1149:i32)
                            n522 = for {
                              N: w1149 -> [_]
                              tunnel: w1148 -> [w1151] mode=indexing
                              tunnel: w1147 -> [w1150] mode=indexing
                              n523 = case shown="True" w1150 {
                                tunnel: w1151 -> [_ w1155]
                                frame False {
                                }
                                frame True {
                                n524 = local read "probe points per region"() -> (w1157:i32[])
                                n525 = Index Array(array=w1157, index=w1155) -> (element=w1156:i32)
                                n526 = flat-sequence {
                                tunnel: w1155 -> [w1162]
                                tunnel: w1156 -> [w1161]
                                tunnel: [w1162] -> w1154
                                tunnel: [w1161] -> w1153
                                tunnel: [w1160] -> w1152
                                tunnel: w1154 -> [w1178]
                                tunnel: w1153 -> [w1175]
                                tunnel: w1152 -> [w1164]
                                frame #0 {
                                n527 = local read "Probe Card Channels"() -> (w1158:i32)
                                n528 = local read "Auto ReCheck"() -> (w1159:bool)
                                n529 = local read "Thresholds:"() -> (w1163:T2)
                                n530 = call "ReCheckStrips.vi"("Probe Card Channels"=w1158, "Auto Re-Check"=w1159, "Thresholds"=w1163, "region in"=w1162, "Number of strips probed"=w1161) -> ("Thresholds copy"=w1160:T16)  [unwired: 6 in]
                                n531 = local write "Thresholds:"(w1160) -> ()
                                }
                                frame #1 {
                                n532 = local read "max scale array"() -> (w1177:i32[])
                                n533 = local read "min scale array"() -> (w1176:i32[])
                                n534 = call "DisplayStriptestData.vi"("min scale array"=w1176, "max scale array"=w1177, "# probed"=w1175, "Display Stats?"=TRUE, "Thresholds"=w1164, "Region"=w1178) -> ("Defects"=w1170:i32[][], "Resistance [MW]"=w1171:cluster{u32, i32, "Array OUT":dbl[]}, "Capacitance [pF]"=w1173:cluster{u32, i32, "Array OUT":dbl[]}, "Current [nA]"=w1172:cluster{u32, i32, "Array OUT":dbl[]}, "Strip Quality Data"=w1169:T15)
                                n535 = Unbundle By Name(w1169) -> ("pass Rate in %"=w1168:dbl, "Bad channel list"=w1167:i32[], "No of bad strips"=w1166:i32, "Number of defects per category"=w1165:i32[])
                                n536 = local write "Current [nA]"(w1172) -> ()
                                n537 = local write "Capacitance [pF]"(w1173) -> ()
                                n538 = local write "Resistance [MW]"(w1171) -> ()
                                n539 = local write "Defects"(w1170) -> ()
                                n540 = local write "% OK:"(w1168) -> ()
                                n541 = local write "Bad Strip List"(w1167) -> ()
                                n542 = local write "# total defects:"(w1166) -> ()
                                n543 = local write "defect type array"(w1165) -> ()
                                }
                                }
                                }
                              }
                            }
                          }
                          frame #1 {
                            n544 = local write "Auto ReCheck"(FALSE) -> ()
                          }
                        }
                      }
                    }
                  }
                }
                n545 = case shown="True" w1113 {
                  tunnel: w1112 -> [w1180 w1187]
                  tunnel: [w1180 w1187] -> w1110
                  frame False {
                  }
                  frame True {
                    n546 = local read "probe points per region"() -> (w1197:i32[])
                    n547 = local read "Region Indices"() -> (w1188:i32[])
                    n548 = local read "max scale array"() -> (w1198:i32[])
                    n549 = local read "min scale array"() -> (w1199:i32[])
                    n550 = local read "Thresholds:"() -> (w1202:T2)
                    n551 = Index Array(array=w1188, index=w1187) -> (element=w1186:i32)
                    n552 = Index Array(array=w1197, index=w1187) -> (element=w1203:i32)
                    n553 = Index Array(array=w1198, index=w1187) -> (element=w1185:i32)
                    n554 = Index Array(array=w1199, index=w1187) -> (element=w1184:i32)
                    n555 = call "DisplayStriptestData.vi"("min scale array"=w1199, "max scale array"=w1198, "# probed"=w1203, "Display Stats?"=TRUE, "Thresholds"=w1202, "Region"=w1186) -> ("Defects"=w1200:i32[][], "Resistance [MW]"=w1194:cluster{u32, i32, "Array OUT":dbl[]}, "Capacitance [pF]"=w1195:cluster{u32, i32, "Array OUT":dbl[]}, "Current [nA]"=w1196:cluster{u32, i32, "Array OUT":dbl[]}, "Strip Quality Data"=w1201:T15)
                    n556 = Increment(x=w1185) -> (x+1=w1182:i32)
                    n557 = Increment(x=w1184) -> (x+1=w1183:i32)
                    n558 = property on="Resistance [MW]" class="WFGraph (strict)"("XScale.Minimum"=w1183) -> ()  [unwired: 2 in, 2 out]
                    n559 = property on="Resistance [MW]" class="WFGraph (strict)"("XScale.Maximum"=w1182) -> ()  [unwired: 2 in, 2 out]
                    n560 = property on="Current [nA]" class="WFGraph (strict)"("XScale.Maximum"=w1182) -> ()  [unwired: 2 in, 2 out]
                    n561 = Unbundle By Name(w1201) -> ("pass Rate in %"=w1191:dbl, "Bad channel list"=w1189:i32[], "No of bad strips"=w1192:i32, "Number of defects per category"=w1190:i32[])
                    n562 = property on="Capacitance [pF]" class="WFGraph (strict)"("XScale.Minimum"=w1183) -> ()  [unwired: 2 in, 2 out]
                    n563 = property on="Defects" class="IntGraph (strict)"("XScale.Minimum"=w1183) -> ()  [unwired: 2 in, 2 out]
                    n564 = local write "Current [nA]"(w1196) -> ()
                    n565 = local write "Capacitance [pF]"(w1195) -> ()
                    n566 = property on="Current [nA]" class="WFGraph (strict)"("XScale.Minimum"=w1183) -> ()  [unwired: 2 in, 2 out]
                    n567 = local write "Resistance [MW]"(w1194) -> ()
                    n568 = local write "Defects"(w1200) -> ()
                    n569 = property on="Capacitance [pF]" class="WFGraph (strict)"("XScale.Maximum"=w1182) -> ()  [unwired: 2 in, 2 out]
                    n570 = Increment(x=w1182) -> (x+1=w1181:i32)
                    n571 = property on="Defects" class="IntGraph (strict)"("XScale.Maximum"=w1181) -> ()  [unwired: 2 in, 2 out]
                    n572 = local write "% OK:"(w1191) -> ()
                    n573 = local write "Bad Strip List"(w1189) -> ()
                    n574 = local write "# total defects:"(w1192) -> ()
                    n575 = local write "defect type array"(w1190) -> ()
                  }
                }
                n576 = Or(x="Save Data", y="Quit w/o saving") -> (x .or. y?=w1114:bool)
              }
              n577 = local write "Save Data"("Auto quit &\nswitch off bias") -> ()
            }
            frame #1 {
              n578 = case shown="False" w1204 {
                frame False {
                  # "supply to standby"
                  n579 = global read "QC_MeasurementSetup.vi" "Striptest Measurement Parameters"() -> (w1216:T7)
                  n580 = Unbundle By Name(w1216) -> ("Bias Supply"=w1205:refnum<class "SupplyControl.lvclass">, "Switching"=w1215:refnum<class "Switching.lvclass">)
                  n581 = local read "Current Bias Voltage [V]"() -> (w1209:dbl)
                  n582 = call-dynamic "MatrixSwitch.vi"("Action"=T5."Reset", "Switching in"=w1215) -> ("error out"=w1214:errorcluster)  [unwired: 7 in, 2 out]
                  n583 = call "SupplyRamp.vi"("error in"=w1214, "Requested Voltage"=0.0, "Step Size"=10.0, "Step Delay"=1000, "Supply IN"=w1205, "Starting Voltage"=w1209) -> ("error out"=w1212:errorcluster, "Supply OUT"=w1211:refnum<class "SupplyControl.lvclass">, "Current Voltage"=w1210:dbl)  [unwired: 2 in, 1 out]
                  n584 = local write "Current Bias Voltage [V]"(w1210) -> ()
                  n585 = call-dynamic "Supply_Stby.vi"("error in (no error)"=w1212, "SupplyControl in"=w1211) -> ()  [unwired: 8 in, 2 out]
                }
                frame True {
                }
              }
            }
            frame #2 {
              n586 = case shown="False" w1219 {
                frame False {
                  n587 = global read "QC_MeasurementSetup.vi" "Striptest Measurement Parameters"() -> (w1221:T7)
                  n588 = Unbundle By Name(w1221) -> ("Arduino"=w1226:refnum<class "ArduinoControl.lvclass">)
                  n589 = local read "Temperature Progression"() -> (w1231:T3)
                  n590 = call "ArduinoRead.vi"("Arduino function"=enum16{"T/RH", "Interlock", "Edgesense"}."T/RH", "ArduinoControl in"=w1226) -> ("error out"=w1232:errorcluster, "Temperature [°C]"=w1223:dbl, "ArduinoControl out"=w1233:refnum<class "ArduinoControl.lvclass">)  [unwired: 4 in, 3 out]
                  "Last Temperature [°C]" <- w1223
                  n591 = call "ArduinoClose.vi"("error in (no error)"=w1232, "ArduinoControl in"=w1233) -> ()  [unwired: 8 in, 2 out]
                  n592 = local read "Run Duration:"() -> (w1228:string)
                  n593 = Unbundle(w1231) -> ("Time Array"=w1229:string[], "Temperature Array [°C]"=w1224:dbl[])  [unwired: 1 out]
                  n594 = Build Array (concatenate)(w1229, w1228) -> (w1227:string[])
                  n595 = Build Array (concatenate)(w1224, w1223) -> (w1222:dbl[])
                  n596 = Bundle(cluster=w1231, "Time Array"=w1227, "Temperature Array [°C]"=w1222) -> (w1230:T3)  [unwired: 1 in]
                  n597 = local write "Temperature Progression"(w1230) -> ()
                }
                frame True {
                }
              }
              n598 = local read "# probed"() -> (w1218:i32)
              n599 = call "SaveJPEG.vi"("Picture No."=w1218, "Test"="Striptest") -> ()  [unwired: 1 in, 2 out]
              n600 = One Button Dialog(message="Please switch bias off NOW and then open\nprobestation enclosure and raise needle.") -> ()  [unwired: 1 in, 1 out]
            }
            frame #3 {
              n601 = One Button Dialog(message="Please ensure detector bias is OFF!") -> ()  [unwired: 1 in, 1 out]
            }
          }
          n602 = case shown="True" w1097 {
            tunnel: [FALSE w1341] -> w1095
            frame False {
            }
            frame True {
              n603 = Two Button Dialog(message="Are you sure you don't want to save the data?", 1:"Quit" ("F button name (\"Cancel\")"), 2:"Save data" ("T button name (\"OK\")")) -> (T button?=w1341:bool)
            }
          }
          n604 = global read "ProbePlanParams.vi" "ProbePlan Parameters IN"() -> (w1094:T10)
          n605 = Unbundle By Name(w1094) -> ("Test ProbePoints.Regions Enabled"=w1092:bool[], "ProbePlan array"=w1091:T11)
          n606 = Array Size(array=w1092) -> (size(s)=w1093:i32)
          n607 = Or(x=w1096, y=w1095) -> (x .or. y?=w1085:bool)
          n608 = case shown="True" w1085 {
            tunnel: w1093 -> [w1241 w1269]
            tunnel: w1092 -> [w1240 w1268]
            tunnel: w1091 -> [_ w1267]
            tunnel: [w1236 w1265] -> w1088
            tunnel: [w1238 w1263] -> w1087
            tunnel: ["" w1260] -> w1086
            frame False {
              n609 = for {
                N: w1241 -> [_]
                tunnel: w1240 -> [w1245] mode=indexing
                tunnel: [w1244] -> w1239 mode=indexing
                tunnel: [w1243] -> w1237 mode=indexing
                i -> [w1242]
                n610 = case shown="True" w1245 {
                  tunnel: [100.0 w1250] -> w1244
                  tunnel: [TRUE w1249] -> w1243
                  tunnel: w1242 -> [_ w1248]
                  frame False {
                  }
                  frame True {
                    n611 = local read "probe points per region"() -> (w1256:i32[])
                    n612 = local read "max scale array"() -> (w1255:i32[])
                    n613 = local read "min scale array"() -> (w1254:i32[])
                    n614 = local read "Thresholds:"() -> (w1258:T2)
                    n615 = Index Array(array=w1256) -> (element=w1252:i32)  [unwired: 1 in]
                    n616 = call "DisplayStriptestData.vi"("min scale array"=w1254, "max scale array"=w1255, "# probed"=w1252, "Display Stats?"=TRUE, "Thresholds"=w1258, "Region"=w1248) -> ("Strip Quality Data"=w1253:T15)  [unwired: 4 out]
                    n617 = Unbundle By Name(w1253) -> ("pass Rate in %"=w1250:dbl)
                    n618 = Greater?(x=w1250, y=98.0) -> (0:w1249:bool)
                  }
                }
              }
              n619 = And Array Elements(Boolean array=w1237) -> (logical AND=w1236:bool)
              n620 = Array Max & Min(array=w1239) -> (min value=w1238:dbl)  [unwired: 3 out]
            }
            frame True {
              n621 = for {
                N: w1269 -> [_]
                tunnel: w1268 -> [w1279] mode=indexing
                tunnel: w1267 -> [w1278] mode=indexing
                tunnel: [w1276] -> w1266 mode=indexing
                tunnel: [w1275] -> w1264 mode=indexing
                tunnel: [w1274] -> w1262
                shift-right: [w1273] -> w1259
                shift-left: _ -> [w1270]
                i -> [w1277]
                n622 = case shown="True" w1279 {
                  tunnel: w1277 -> [_ w1292]
                  tunnel: w1278 -> [_ w1291]
                  tunnel: [TRUE w1288] -> w1276
                  tunnel: [100.0 w1286] -> w1275
                  tunnel: [w1280 w1285] -> w1274
                  tunnel: [w1280 w1284] -> w1271
                  frame False {
                    w1280 = ""
                  }
                  frame True {
                    n623 = Unbundle By Name(w1291) -> ("Region"=w1290:string)
                    n624 = flat-sequence {
                      tunnel: w1292 -> [w1316]
                      tunnel: w1290 -> [w1293]
                      tunnel: [w1316] -> w1289
                      tunnel: [w1317] -> w1287
                      tunnel: [w1295] -> w1285
                      tunnel: [w1294] -> w1284
                      tunnel: [w1293] -> w1283
                      tunnel: w1289 -> [w1328]
                      tunnel: [w1330] -> w1288
                      tunnel: w1287 -> [w1326]
                      tunnel: [w1327] -> w1286
                      tunnel: w1283 -> [w1325]
                      frame #0 {
                        w1310 = T17."Read Array" ("Action")
                        n625 = Concatenate Strings("Saving data for " ("string"), w1293) -> (w1323:string)
                        n626 = local write "Status:"(w1323) -> ()
                        n627 = call "MultiRegionData.vi"("Action"=w1310, "Array No."=4, "Region index"=w1316) -> ("Array OUT"=w1308:dbl[])  [unwired: 3 in, 1 out]
                        n628 = Multiply(x=w1308, y=0.001) -> (x*y=w1307:dbl[])
                        n629 = call "MultiRegionData.vi"("Action"=w1310, "Array No."=0, "Region index"=w1316) -> ("Array OUT"=w1303:dbl[])  [unwired: 3 in, 1 out]
                        n630 = call "MultiRegionData.vi"("Action"=w1310, "Array No."=1, "Region index"=w1316) -> ("Array OUT"=w1304:dbl[])  [unwired: 3 in, 1 out]
                        n631 = call "MultiRegionData.vi"("Action"=w1310, "Array No."=3, "Region index"=w1316) -> ("Array OUT"=w1306:dbl[])  [unwired: 3 in, 1 out]
                        n632 = local read "Temperature Progression"() -> (w1298:T3)
                        n633 = call "MultiRegionData.vi"("Array No."=2, "Region index"=w1316) -> ("Array OUT"=w1305:dbl[])  [unwired: 4 in, 1 out]
                        n634 = Build Array(w1303, w1304, w1305, w1306, w1307) -> (w1302:dbl[][])
                        n635 = Transpose 2D Array(2D array=w1302) -> (transposed array=w1301:dbl[][])
                        n636 = local read "probe points per region"() -> (w1324:i32[])
                        n637 = Unbundle By Name(w1298) -> ("Temperature Array [°C]"=w1297:dbl[], "Humidity Array [RH %]"=w1296:dbl[])
                        n638 = call <vilib>:"Std Deviation and Variance.vi"("X"=w1297) -> ("mean"=w1300:dbl)  [unwired: 1 in, 2 out]
                        n639 = call <vilib>:"Std Deviation and Variance.vi"("X"=w1296) -> ("mean"=w1299:dbl)  [unwired: 1 in, 2 out]
                        n640 = Index Array(array=w1324, index=w1316) -> (element=w1319:i32)
                        n641 = call "SaveDataFile.vi"("Data Array"=w1301, "Temperature"=w1300, "Humidity"=w1299, "no. of arrays"=5, "Actual array lengths"=w1319, "Array Titles"="ProbeplanIndex Current PinholeFlag Capacitance Resistance", "Strip Segment"=w1293, "Arrays format"="%016.6f") -> ("Filename OUT"=w1294:string, "Pathname OUT"=w1295:string, "Path + Filename OUT"=w1317:string)  [unwired: 4 in, 1 out]
                      }
                      frame #1 {
                        n642 = local read "probe points per region"() -> (w1337:i32[])
                        n643 = local read "max scale array"() -> (w1336:i32[])
                        n644 = local read "min scale array"() -> (w1335:i32[])
                        n645 = local read "Thresholds:"() -> (w1339:T2)
                        n646 = Index Array(array=w1337, index=w1328) -> (element=w1329:i32)
                        n647 = call "DisplayStriptestData.vi"("min scale array"=w1335, "max scale array"=w1336, "# probed"=w1329, "Display Stats?"=TRUE, "Thresholds"=w1339, "Region"=w1328) -> ("Strip Quality Data"=w1334:T15)  [unwired: 4 out]
                        n648 = Unbundle By Name(w1334) -> ("pass Rate in %"=w1327:dbl, "Bad channel list"=w1333:i32[], "No of bad strips"=w1332:i32, "Defect description list"=w1331:i32[])
                        n649 = call "CreateDefectFile.vi"("Segment:"=w1325, "Pass rate"=w1327, "Defect description list"=w1331, "Bad channel array"=w1333, "No of bad strips"=w1332, "Filename IN"=w1326) -> ("passed"=w1330:bool)  [unwired: 3 in, 2 out]
                      }
                    }
                  }
                }
                n650 = call <vilib>:"Space Constant.vi"() -> ("String"=w1272:string)
                n651 = Concatenate Strings(w1270, w1272, w1271) -> (w1273:string)
              }
              n652 = Array Max & Min(array=w1264) -> (min value=w1263:dbl)  [unwired: 3 out]
              n653 = And Array Elements(Boolean array=w1266) -> (logical AND=w1265:bool)
              "Module failed/passed" <- w1265
              n654 = call <vilib>:"Space Constant.vi"() -> ("String"=w1261:string)
              n655 = Concatenate Strings(w1262, w1261, w1259) -> (w1260:string)
            }
          }
          n656 = local read "Temperature Progression"() -> (w1084:T3)
          n657 = Unbundle By Name(w1084) -> ("Temperature Array [°C]"=w1082:dbl[], "Humidity Array [RH %]"=w1083:dbl[])
          n658 = call <vilib>:"Std Deviation and Variance.vi"("X"=w1082) -> ("standard deviation"=w1076:dbl)  [unwired: 1 in, 2 out]
          n659 = call <vilib>:"Std Deviation and Variance.vi"("X"=w1083) -> ("standard deviation"=w1075:dbl)  [unwired: 1 in, 2 out]
          n660 = Greater?(x=w1076, y=5) -> (0:w1073:bool)
          n661 = Greater?(x=w1075, y=10) -> (0:w1074:bool)
          n662 = Select(t="large temperature fluctuations", s=w1073, f=w1079) -> (s? t:f=w1070:string)
          n663 = Select(t="large humidity fluctuations", s=w1074, f=w1079) -> (s? t:f=w1071:string)
          n664 = Concatenate Strings(w1070, "\t", w1071) -> (w1069:string)
          n665 = call "WriteLogFile.vi"("Automatic warning"=w1069, "Data File"=w1086, "DUT passed?"=w1088, "Value TechSpec criteria"=w1087, "Files saved?"=w1085) -> ()  [unwired: 6 in, 1 out]
        }
      }
    }
  }
